vi "Musicplayerversuch_mit_Liste.vi"() -> ()   [LabVIEW 2010]
uses:
  <vilib>/sound2/lvsound2.llb/Sound File Position.ctl
  <vilib>/sound2/lvsound2.llb/Sampling Mode.ctl
  <vilib>/Utility/miscctls.llb/LVRowAndColumnTypeDef.ctl
  <vilib>/Utility/cursorutil.llb/Set Cursor (Icon Pict).vi
  <vilib>/gmath/NI_Gmath.lvlib
  <vilib>/Utility/miscctls.llb/LVKeyTypeDef.ctl
  <vilib>/gmath/statdist.llb/Uniform (Discrete) Random.vi
  <vilib>/Utility/inputDevices.llb/closeKeyboard.vi
  <vilib>/Utility/inputDevices.llb/keyboardAcquire.vi
  <vilib>/sound2/lvsound2.llb/Sound File Read Open.vi
  <vilib>/sound2/lvsound2.llb/Sound File Info (path).vi
  <vilib>/sound2/lvsound2.llb/Sound Output Write (DBL).vi
  <vilib>/sound2/lvsound2.llb/Sound Output Set Volume (Single).vi
  <vilib>/sound2/lvsound2.llb/Sound File Read (DBL).vi
  <vilib>/Utility/file.llb/Write To Spreadsheet File (string).vi
  <vilib>/Utility/file.llb/Read From Spreadsheet File (string).vi
panel:
  in  "plalist umschalten":bool
  in  "Playlist 2":i32(listbox) caption="Playlist"
  in  "nach diesem lied stoppen":bool caption="nach diesem Titel stoppen"
  out "Lieder:":dbl
  in  "shortcut's":bool caption="Kürzel"
  in  "min.Sound":bool caption="min.Lautstärke"
  in  "max.Sound":bool caption="max.Lautsärke"
  in  "counter":bool
  in  "Volume":i64(slide) caption="Lautstärke" min=0 max=100 scale=0.0..100.0
  in  "danach Playlist Start":bool
  in  "Einzeiln":bool
  in  "Hinzufügen":bool
  in  "Musicauswählen":bool
  out "Musicanzeige":string
  in  "Deutsch?":bool
  out "ausgewählt":bool
  out "Zeilezumeinfügen":i32
  in  "Playlist 3":string[][](table)
  in  "veränderung":bool
  out "=":dbl
  in  "Farbfeld":u32(colorbox)
  out "Cluster":T1
  in  "zu spielende Lieder:":dbl
  in  "gespielte Lieder:":dbl
  in  "Gespielte Lieder tabelle":string[][](table)
  in  "icon 2":u16(ring) caption="Symbol"
  in  "icon":u16(ring)=13 caption="Symbol"
  out "Fehler (Ausgang)":errorcluster
  in  "go to line?":bool
  in  "Column":i32
  in  "Row":i32
  in  "Pfad":path
  out "Spalte":dbl
  in  "Seite":dbl
  out "Gelesener Pfad":string
  in  "Language":enum32{"Englisch", "German"}(radio)
  in  "optionen":bool
  in  "Sperren":bool
  out "dup path":path
  in  "anaus":bool
  out "Sicherheitsdati":path
  in  "Start?":bool
  in  "OK Passwort":bool
  out "Text":string="Bitte den Aktivierungscode eingeben."
  out "OK-Schaltfläche":bool
  in  "von, bis":bool
  in  "to":dbl=1.0 caption="bis" min=1.0
  in  "from":dbl=1.0 caption="von" min=1.0
  in  "liste löschen":bool
  in  "gehe zur zeile kn.":bool
  in  "gehe zur zeile":dbl=1.0 min=1.0
  in  "Realtime?":bool
  in  "device ID":u32 caption="Device-ID"
  in  "background":bool
  in  "Info":bool
  in  "Hilfe":bool
  in  "Schließen.":bool
  in  "Pause":bool
  in  "Wiederholen":bool
  in  "Stop":bool
  in  "Play":bool
  out "Verdekung":bool
  in  "Playlist":string[][](table)
  out "Play?":bool
  in  "playlist laden":bool
  in  "playlist speichern":bool
  out "Einzeiln 2":bool
  in  "nächtes lied":bool
  in  "zufall":bool
  out "Lerrerpad?":bool
  out "end of file?":bool caption="Dateiende?"
  in  "zeile entfernen":bool
  out "Stop?":bool
  in  "Wiederholen?":bool
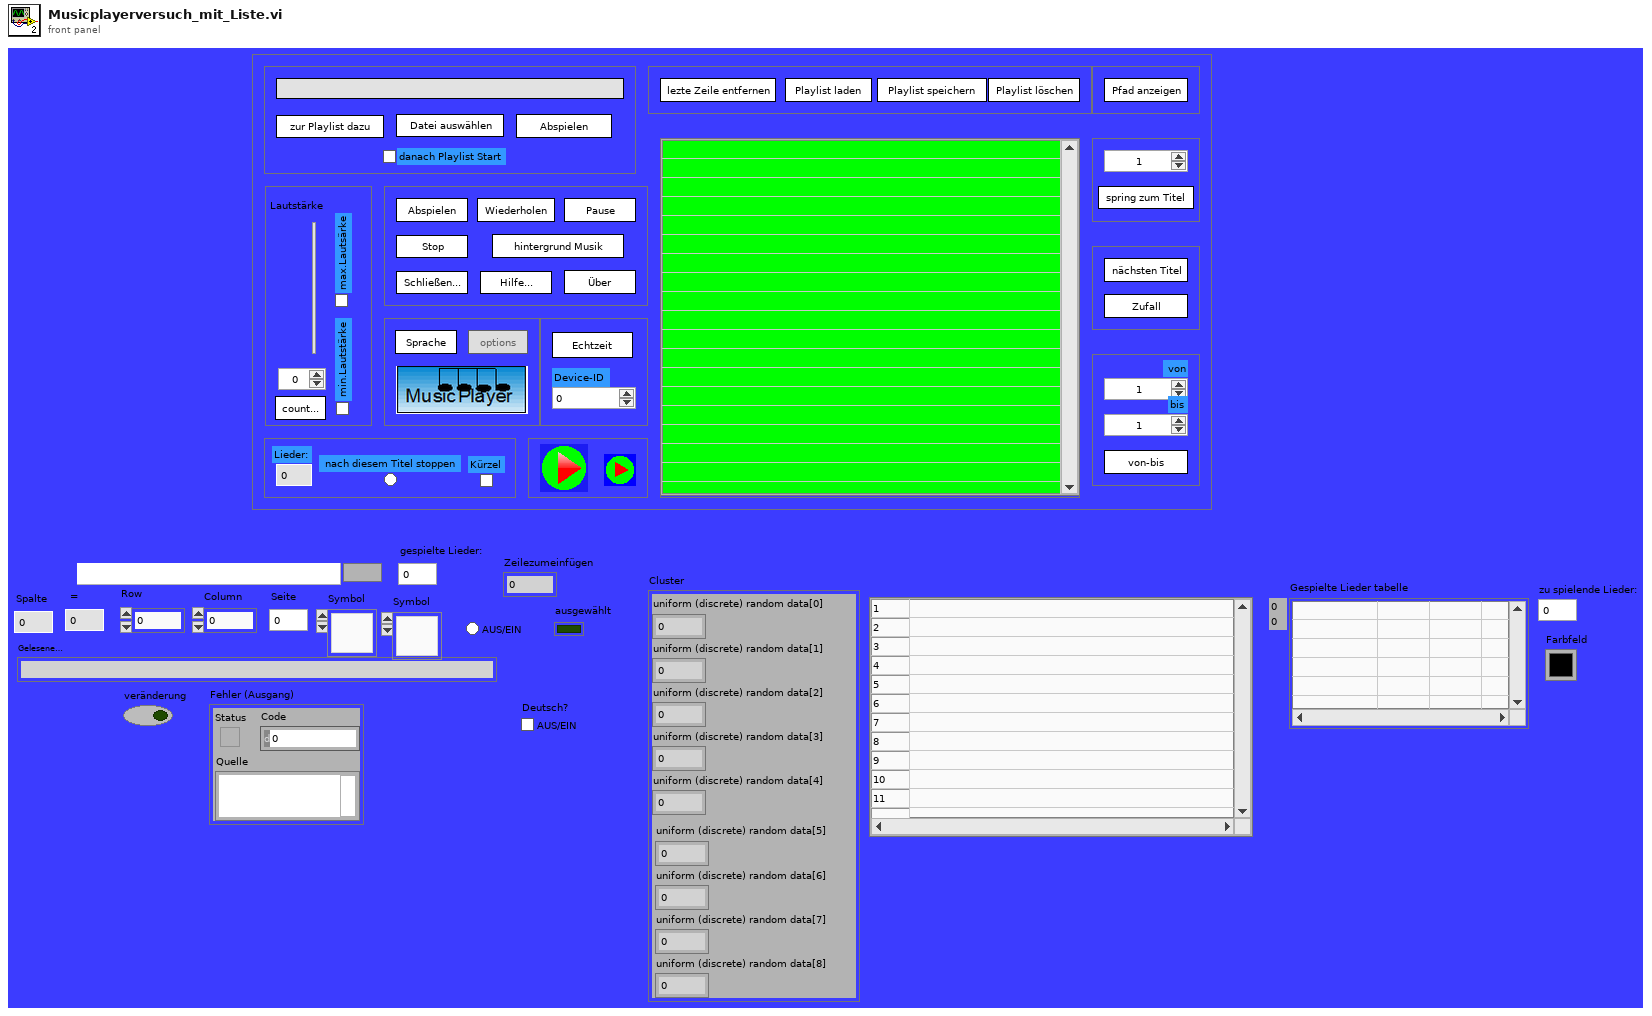
[diagram p1: front panel]
types:
  T1 = cluster{"uniform (discrete) random data[0]":i32, "uniform (discrete) random data[1]":i32, "uniform (discrete) random data[2]":i32, "uniform (discrete) random data[3]":i32, "uniform (discrete) random data[4]":i32, "uniform (discrete) random data[5]":i32, "uniform (discrete) random data[6]":i32, "uniform (discrete) random data[7]":i32, "uniform (discrete) random data[8]":i32}
  T2 = enum16{"open", "replace", "create", "open or create", "replace or create", "replace or create with confirmation"}
  T3 = typedef "LVKeyTypeDef.ctl" = cluster{"Focus":bool, "Control":bool, "Shift":bool, "Key":string}
  T4 = enum16{"0", "1", "2", "3", "4", "5", "6", "7", "8", "9", "A", "B", "C", "D", "E", "F", "G", "H", "I", "J", "K", "L", "M", "N", "O", "P", "Q", "R", "S", "T", "U", "V", "W", "X", "Y", "Z", "F1", "F2", "F3", "F4", "F5", "F6", "F7", "F8", "F9", "F10", "F11", "F12", "F13", "F14", "F15", "ADD", "BACK", "BACKSLASH", "CAPITAL", "COMMA", "DECIMAL", "DELETE", "DIVIDE", "DOWN", "END", "EQUALS", "ESCAPE", "GRAVE (`)", "HOME", "INSERT", "LBRACKET", "LCONTROL", "LEFT", "L ALT", "LSHIFT", "LWIN", "MINUS", "MULTIPLY", "NEXT", "NUMLOCK", "NUMPAD_0", "NUMPAD_1", "NUMPAD_2", "NUMPAD_3", "NUMPAD_4", "NUMPAD_5", "NUMPAD_6", "NUMPAD_7", "NUMPAD_8", "NUMPAD_9", "PAUSE", "PERIOD", "PRIOR (PG UP)", "RBRACKET", "RCONTROL", "RETURN", "RIGHT", "R ALT", "RSHIFT", "RWIN", "SCROLL", "SEMICOLON", "SLASH", "SPACE", "SUBTRACT", "TAB", "UP", "ENTER (num pad)", "' (quote)"}
  T5 = typedef "LVRowAndColumnTypeDef.ctl" = cluster{"Row":i32, "Column":i32}
  T6 = typedef "Sampling Mode.ctl" = i32
  T7 = typedef "Sound Data Format.ctl" = cluster{"sample rate (S/s)":dbl, "number of channels":i32, "bits per sample":i32}
  T8 = typedef "Sound File Refnum.ctl" = refnum<file>
  T9 = typedef "Sound Output Task ID.ctl" = u32
  T10 = typedef "Sound File Position.ctl" = u16
  T11 = enum16{"0", "1", "2", "3", "4", "5", "6", "7", "8", "9", "A", "B", "C", "D", "E", "F", "G", "H", "I", "J", "K", "L", "M", "N", "O", "P", "Q", "R", "S", "T", "U", "V", "W", "X", "Y", "Z", "F1", "F2", "F3", "F4", "F5", "F6", "F7", "F8", "F9", "F10", "F11", "F12", "F13", "F14", "F15", "ADD", "BACK", "BACKSLASH", "CAPITAL", "COMMA", "DECIMAL", "DELETE", "DIVIDE", "DOWN", "END", "EQUALS", "ESCAPE", "GRAVE (`)", "HOME", "INSERT", "LBRACKET", "LCONTROL", "LEFT", "L ALT", "LSHIFT", "LWIN", "MINUS", "MULTIPLY", "NEXT", "NUMLOCK", "NUMPAD_0", "NUMPAD_1", "NUMPAD_2", "NUMPAD_3", "NUMPAD_4", "NUMPAD_5", "NUMPAD_6", "NUMPAD_7", "NUMPAD_8", "NUMPAD_9", "PAUSE", "PERIOD", "PRIOR (PG UP)", "RBRACKET", "RCONTROL", "RETURN", "RIGHT", "R ALT", "RSHIFT", "RWIN", "SCROLL", "SEMICOLON", "SLASH", "SPACE", "SUBTRACT", "TAB", "UP", "ENTER (num pad)", "' (quote)"}[]
  T12 = cluster{"keys pressed[0]":enum16{"0", "1", "2", "3", "4", "5", "6", "7", "8", "9", "A", "B", "C", "D", "E", "F", "G", "H", "I", "J", "K", "L", "M", "N", "O", "P", "Q", "R", "S", "T", "U", "V", "W", "X", "Y", "Z", "F1", "F2", "F3", "F4", "F5", "F6", "F7", "F8", "F9", "F10", "F11", "F12", "F13", "F14", "F15", "ADD", "BACK", "BACKSLASH", "CAPITAL", "COMMA", "DECIMAL", "DELETE", "DIVIDE", "DOWN", "END", "EQUALS", "ESCAPE", "GRAVE (`)", "HOME", "INSERT", "LBRACKET", "LCONTROL", "LEFT", "L ALT", "LSHIFT", "LWIN", "MINUS", "MULTIPLY", "NEXT", "NUMLOCK", "NUMPAD_0", "NUMPAD_1", "NUMPAD_2", "NUMPAD_3", "NUMPAD_4", "NUMPAD_5", "NUMPAD_6", "NUMPAD_7", "NUMPAD_8", "NUMPAD_9", "PAUSE", "PERIOD", "PRIOR (PG UP)", "RBRACKET", "RCONTROL", "RETURN", "RIGHT", "R ALT", "RSHIFT", "RWIN", "SCROLL", "SEMICOLON", "SLASH", "SPACE", "SUBTRACT", "TAB", "UP", "ENTER (num pad)", "' (quote)"}, "keys pressed[1]":enum16{"0", "1", "2", "3", "4", "5", "6", "7", "8", "9", "A", "B", "C", "D", "E", "F", "G", "H", "I", "J", "K", "L", "M", "N", "O", "P", "Q", "R", "S", "T", "U", "V", "W", "X", "Y", "Z", "F1", "F2", "F3", "F4", "F5", "F6", "F7", "F8", "F9", "F10", "F11", "F12", "F13", "F14", "F15", "ADD", "BACK", "BACKSLASH", "CAPITAL", "COMMA", "DECIMAL", "DELETE", "DIVIDE", "DOWN", "END", "EQUALS", "ESCAPE", "GRAVE (`)", "HOME", "INSERT", "LBRACKET", "LCONTROL", "LEFT", "L ALT", "LSHIFT", "LWIN", "MINUS", "MULTIPLY", "NEXT", "NUMLOCK", "NUMPAD_0", "NUMPAD_1", "NUMPAD_2", "NUMPAD_3", "NUMPAD_4", "NUMPAD_5", "NUMPAD_6", "NUMPAD_7", "NUMPAD_8", "NUMPAD_9", "PAUSE", "PERIOD", "PRIOR (PG UP)", "RBRACKET", "RCONTROL", "RETURN", "RIGHT", "R ALT", "RSHIFT", "RWIN", "SCROLL", "SEMICOLON", "SLASH", "SPACE", "SUBTRACT", "TAB", "UP", "ENTER (num pad)", "' (quote)"}, "keys pressed[2]":enum16{"0", "1", "2", "3", "4", "5", "6", "7", "8", "9", "A", "B", "C", "D", "E", "F", "G", "H", "I", "J", "K", "L", "M", "N", "O", "P", "Q", "R", "S", "T", "U", "V", "W", "X", "Y", "Z", "F1", "F2", "F3", "F4", "F5", "F6", "F7", "F8", "F9", "F10", "F11", "F12", "F13", "F14", "F15", "ADD", "BACK", "BACKSLASH", "CAPITAL", "COMMA", "DECIMAL", "DELETE", "DIVIDE", "DOWN", "END", "EQUALS", "ESCAPE", "GRAVE (`)", "HOME", "INSERT", "LBRACKET", "LCONTROL", "LEFT", "L ALT", "LSHIFT", "LWIN", "MINUS", "MULTIPLY", "NEXT", "NUMLOCK", "NUMPAD_0", "NUMPAD_1", "NUMPAD_2", "NUMPAD_3", "NUMPAD_4", "NUMPAD_5", "NUMPAD_6", "NUMPAD_7", "NUMPAD_8", "NUMPAD_9", "PAUSE", "PERIOD", "PRIOR (PG UP)", "RBRACKET", "RCONTROL", "RETURN", "RIGHT", "R ALT", "RSHIFT", "RWIN", "SCROLL", "SEMICOLON", "SLASH", "SPACE", "SUBTRACT", "TAB", "UP", "ENTER (num pad)", "' (quote)"}, "keys pressed[3]":enum16{"0", "1", "2", "3", "4", "5", "6", "7", "8", "9", "A", "B", "C", "D", "E", "F", "G", "H", "I", "J", "K", "L", "M", "N", "O", "P", "Q", "R", "S", "T", "U", "V", "W", "X", "Y", "Z", "F1", "F2", "F3", "F4", "F5", "F6", "F7", "F8", "F9", "F10", "F11", "F12", "F13", "F14", "F15", "ADD", "BACK", "BACKSLASH", "CAPITAL", "COMMA", "DECIMAL", "DELETE", "DIVIDE", "DOWN", "END", "EQUALS", "ESCAPE", "GRAVE (`)", "HOME", "INSERT", "LBRACKET", "LCONTROL", "LEFT", "L ALT", "LSHIFT", "LWIN", "MINUS", "MULTIPLY", "NEXT", "NUMLOCK", "NUMPAD_0", "NUMPAD_1", "NUMPAD_2", "NUMPAD_3", "NUMPAD_4", "NUMPAD_5", "NUMPAD_6", "NUMPAD_7", "NUMPAD_8", "NUMPAD_9", "PAUSE", "PERIOD", "PRIOR (PG UP)", "RBRACKET", "RCONTROL", "RETURN", "RIGHT", "R ALT", "RSHIFT", "RWIN", "SCROLL", "SEMICOLON", "SLASH", "SPACE", "SUBTRACT", "TAB", "UP", "ENTER (num pad)", "' (quote)"}, "keys pressed[4]":enum16{"0", "1", "2", "3", "4", "5", "6", "7", "8", "9", "A", "B", "C", "D", "E", "F", "G", "H", "I", "J", "K", "L", "M", "N", "O", "P", "Q", "R", "S", "T", "U", "V", "W", "X", "Y", "Z", "F1", "F2", "F3", "F4", "F5", "F6", "F7", "F8", "F9", "F10", "F11", "F12", "F13", "F14", "F15", "ADD", "BACK", "BACKSLASH", "CAPITAL", "COMMA", "DECIMAL", "DELETE", "DIVIDE", "DOWN", "END", "EQUALS", "ESCAPE", "GRAVE (`)", "HOME", "INSERT", "LBRACKET", "LCONTROL", "LEFT", "L ALT", "LSHIFT", "LWIN", "MINUS", "MULTIPLY", "NEXT", "NUMLOCK", "NUMPAD_0", "NUMPAD_1", "NUMPAD_2", "NUMPAD_3", "NUMPAD_4", "NUMPAD_5", "NUMPAD_6", "NUMPAD_7", "NUMPAD_8", "NUMPAD_9", "PAUSE", "PERIOD", "PRIOR (PG UP)", "RBRACKET", "RCONTROL", "RETURN", "RIGHT", "R ALT", "RSHIFT", "RWIN", "SCROLL", "SEMICOLON", "SLASH", "SPACE", "SUBTRACT", "TAB", "UP", "ENTER (num pad)", "' (quote)"}, "keys pressed[5]":enum16{"0", "1", "2", "3", "4", "5", "6", "7", "8", "9", "A", "B", "C", "D", "E", "F", "G", "H", "I", "J", "K", "L", "M", "N", "O", "P", "Q", "R", "S", "T", "U", "V", "W", "X", "Y", "Z", "F1", "F2", "F3", "F4", "F5", "F6", "F7", "F8", "F9", "F10", "F11", "F12", "F13", "F14", "F15", "ADD", "BACK", "BACKSLASH", "CAPITAL", "COMMA", "DECIMAL", "DELETE", "DIVIDE", "DOWN", "END", "EQUALS", "ESCAPE", "GRAVE (`)", "HOME", "INSERT", "LBRACKET", "LCONTROL", "LEFT", "L ALT", "LSHIFT", "LWIN", "MINUS", "MULTIPLY", "NEXT", "NUMLOCK", "NUMPAD_0", "NUMPAD_1", "NUMPAD_2", "NUMPAD_3", "NUMPAD_4", "NUMPAD_5", "NUMPAD_6", "NUMPAD_7", "NUMPAD_8", "NUMPAD_9", "PAUSE", "PERIOD", "PRIOR (PG UP)", "RBRACKET", "RCONTROL", "RETURN", "RIGHT", "R ALT", "RSHIFT", "RWIN", "SCROLL", "SEMICOLON", "SLASH", "SPACE", "SUBTRACT", "TAB", "UP", "ENTER (num pad)", "' (quote)"}, "keys pressed[6]":enum16{"0", "1", "2", "3", "4", "5", "6", "7", "8", "9", "A", "B", "C", "D", "E", "F", "G", "H", "I", "J", "K", "L", "M", "N", "O", "P", "Q", "R", "S", "T", "U", "V", "W", "X", "Y", "Z", "F1", "F2", "F3", "F4", "F5", "F6", "F7", "F8", "F9", "F10", "F11", "F12", "F13", "F14", "F15", "ADD", "BACK", "BACKSLASH", "CAPITAL", "COMMA", "DECIMAL", "DELETE", "DIVIDE", "DOWN", "END", "EQUALS", "ESCAPE", "GRAVE (`)", "HOME", "INSERT", "LBRACKET", "LCONTROL", "LEFT", "L ALT", "LSHIFT", "LWIN", "MINUS", "MULTIPLY", "NEXT", "NUMLOCK", "NUMPAD_0", "NUMPAD_1", "NUMPAD_2", "NUMPAD_3", "NUMPAD_4", "NUMPAD_5", "NUMPAD_6", "NUMPAD_7", "NUMPAD_8", "NUMPAD_9", "PAUSE", "PERIOD", "PRIOR (PG UP)", "RBRACKET", "RCONTROL", "RETURN", "RIGHT", "R ALT", "RSHIFT", "RWIN", "SCROLL", "SEMICOLON", "SLASH", "SPACE", "SUBTRACT", "TAB", "UP", "ENTER (num pad)", "' (quote)"}, "keys pressed[7]":enum16{"0", "1", "2", "3", "4", "5", "6", "7", "8", "9", "A", "B", "C", "D", "E", "F", "G", "H", "I", "J", "K", "L", "M", "N", "O", "P", "Q", "R", "S", "T", "U", "V", "W", "X", "Y", "Z", "F1", "F2", "F3", "F4", "F5", "F6", "F7", "F8", "F9", "F10", "F11", "F12", "F13", "F14", "F15", "ADD", "BACK", "BACKSLASH", "CAPITAL", "COMMA", "DECIMAL", "DELETE", "DIVIDE", "DOWN", "END", "EQUALS", "ESCAPE", "GRAVE (`)", "HOME", "INSERT", "LBRACKET", "LCONTROL", "LEFT", "L ALT", "LSHIFT", "LWIN", "MINUS", "MULTIPLY", "NEXT", "NUMLOCK", "NUMPAD_0", "NUMPAD_1", "NUMPAD_2", "NUMPAD_3", "NUMPAD_4", "NUMPAD_5", "NUMPAD_6", "NUMPAD_7", "NUMPAD_8", "NUMPAD_9", "PAUSE", "PERIOD", "PRIOR (PG UP)", "RBRACKET", "RCONTROL", "RETURN", "RIGHT", "R ALT", "RSHIFT", "RWIN", "SCROLL", "SEMICOLON", "SLASH", "SPACE", "SUBTRACT", "TAB", "UP", "ENTER (num pad)", "' (quote)"}, "keys pressed[8]":enum16{"0", "1", "2", "3", "4", "5", "6", "7", "8", "9", "A", "B", "C", "D", "E", "F", "G", "H", "I", "J", "K", "L", "M", "N", "O", "P", "Q", "R", "S", "T", "U", "V", "W", "X", "Y", "Z", "F1", "F2", "F3", "F4", "F5", "F6", "F7", "F8", "F9", "F10", "F11", "F12", "F13", "F14", "F15", "ADD", "BACK", "BACKSLASH", "CAPITAL", "COMMA", "DECIMAL", "DELETE", "DIVIDE", "DOWN", "END", "EQUALS", "ESCAPE", "GRAVE (`)", "HOME", "INSERT", "LBRACKET", "LCONTROL", "LEFT", "L ALT", "LSHIFT", "LWIN", "MINUS", "MULTIPLY", "NEXT", "NUMLOCK", "NUMPAD_0", "NUMPAD_1", "NUMPAD_2", "NUMPAD_3", "NUMPAD_4", "NUMPAD_5", "NUMPAD_6", "NUMPAD_7", "NUMPAD_8", "NUMPAD_9", "PAUSE", "PERIOD", "PRIOR (PG UP)", "RBRACKET", "RCONTROL", "RETURN", "RIGHT", "R ALT", "RSHIFT", "RWIN", "SCROLL", "SEMICOLON", "SLASH", "SPACE", "SUBTRACT", "TAB", "UP", "ENTER (num pad)", "' (quote)"}}
  T13 = enum16{"Left Button", "Center Button", "Right Button", "Window Close"}
  T14 = typedef "eventvkey.ctl" = enum16{"ASCII", "Enter", "Return", "Shift", "Ctrl", "Alt", "Cmd", "Opt", "Caps", "NumLock", "Clear", "Break", "Up", "Down", "Left", "Right", "Insert", "Delete", "Home", "End", "PageUp", "PageDown", "Escape", "Help", "Pause", "ScrollLock", "F1", "F2", "F3", "F4", "F5", "F6", "F7", "F8", "F9", "F10", "F11", "F12", "F13", "F14", "F15", "F16", "F17", "F18", "F19", "F20", "F21", "F22", "F23", "F24", "Play", "VolumeUp", "VolumeDown", "Mute", "Two Byte Char"}
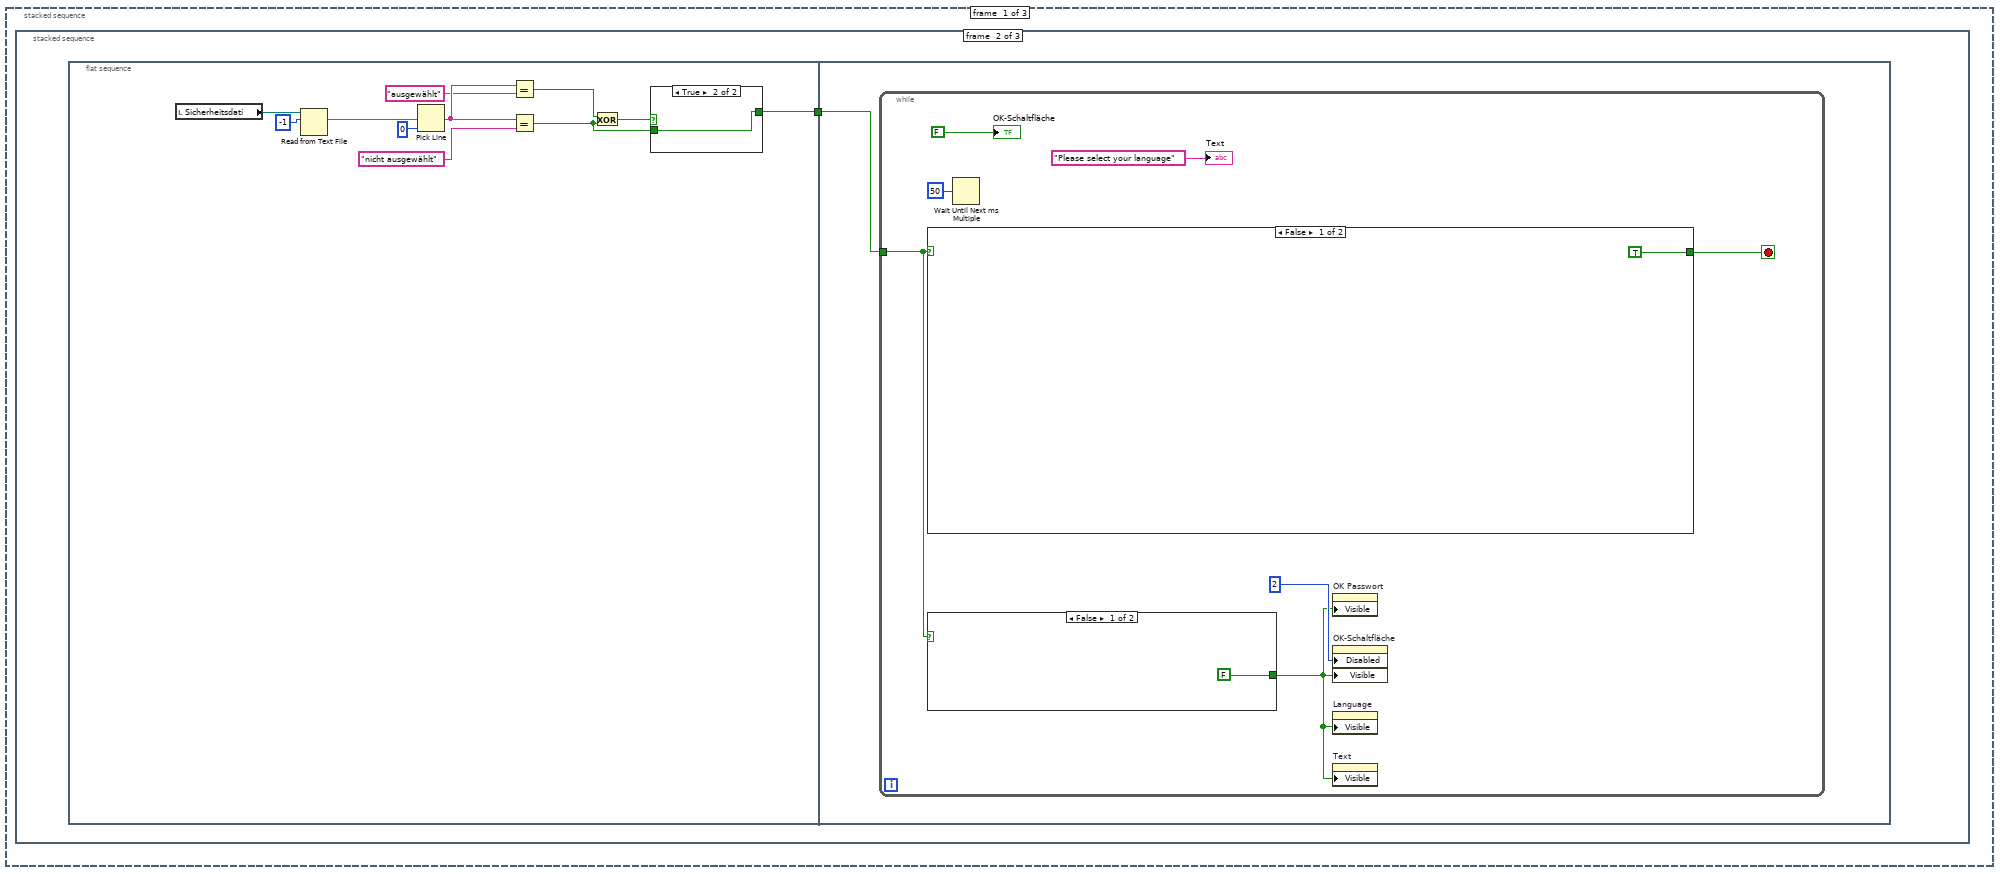
[diagram p2: hidden frame]
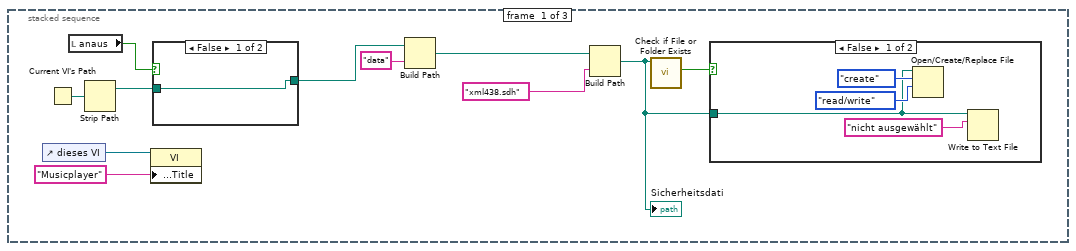
[diagram p3: hidden frame]
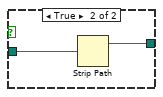
[diagram p4: hidden frame]
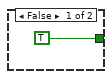
[diagram p6: hidden frame]
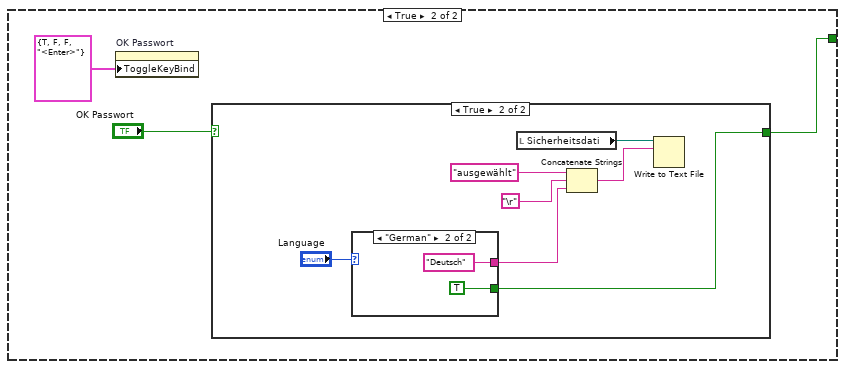
[diagram p7: hidden frame]
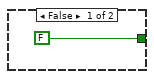
[diagram p8: hidden frame]
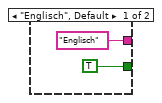
[diagram p9: hidden frame]
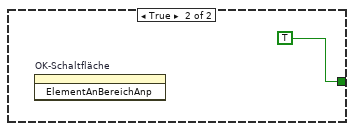
[diagram p10: hidden frame]
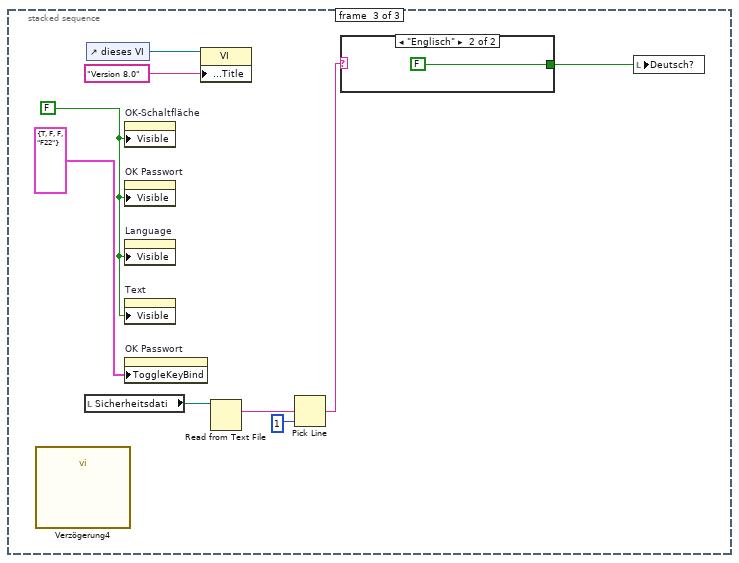
[diagram p11: hidden frame]
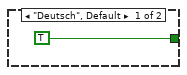
[diagram p12: hidden frame]
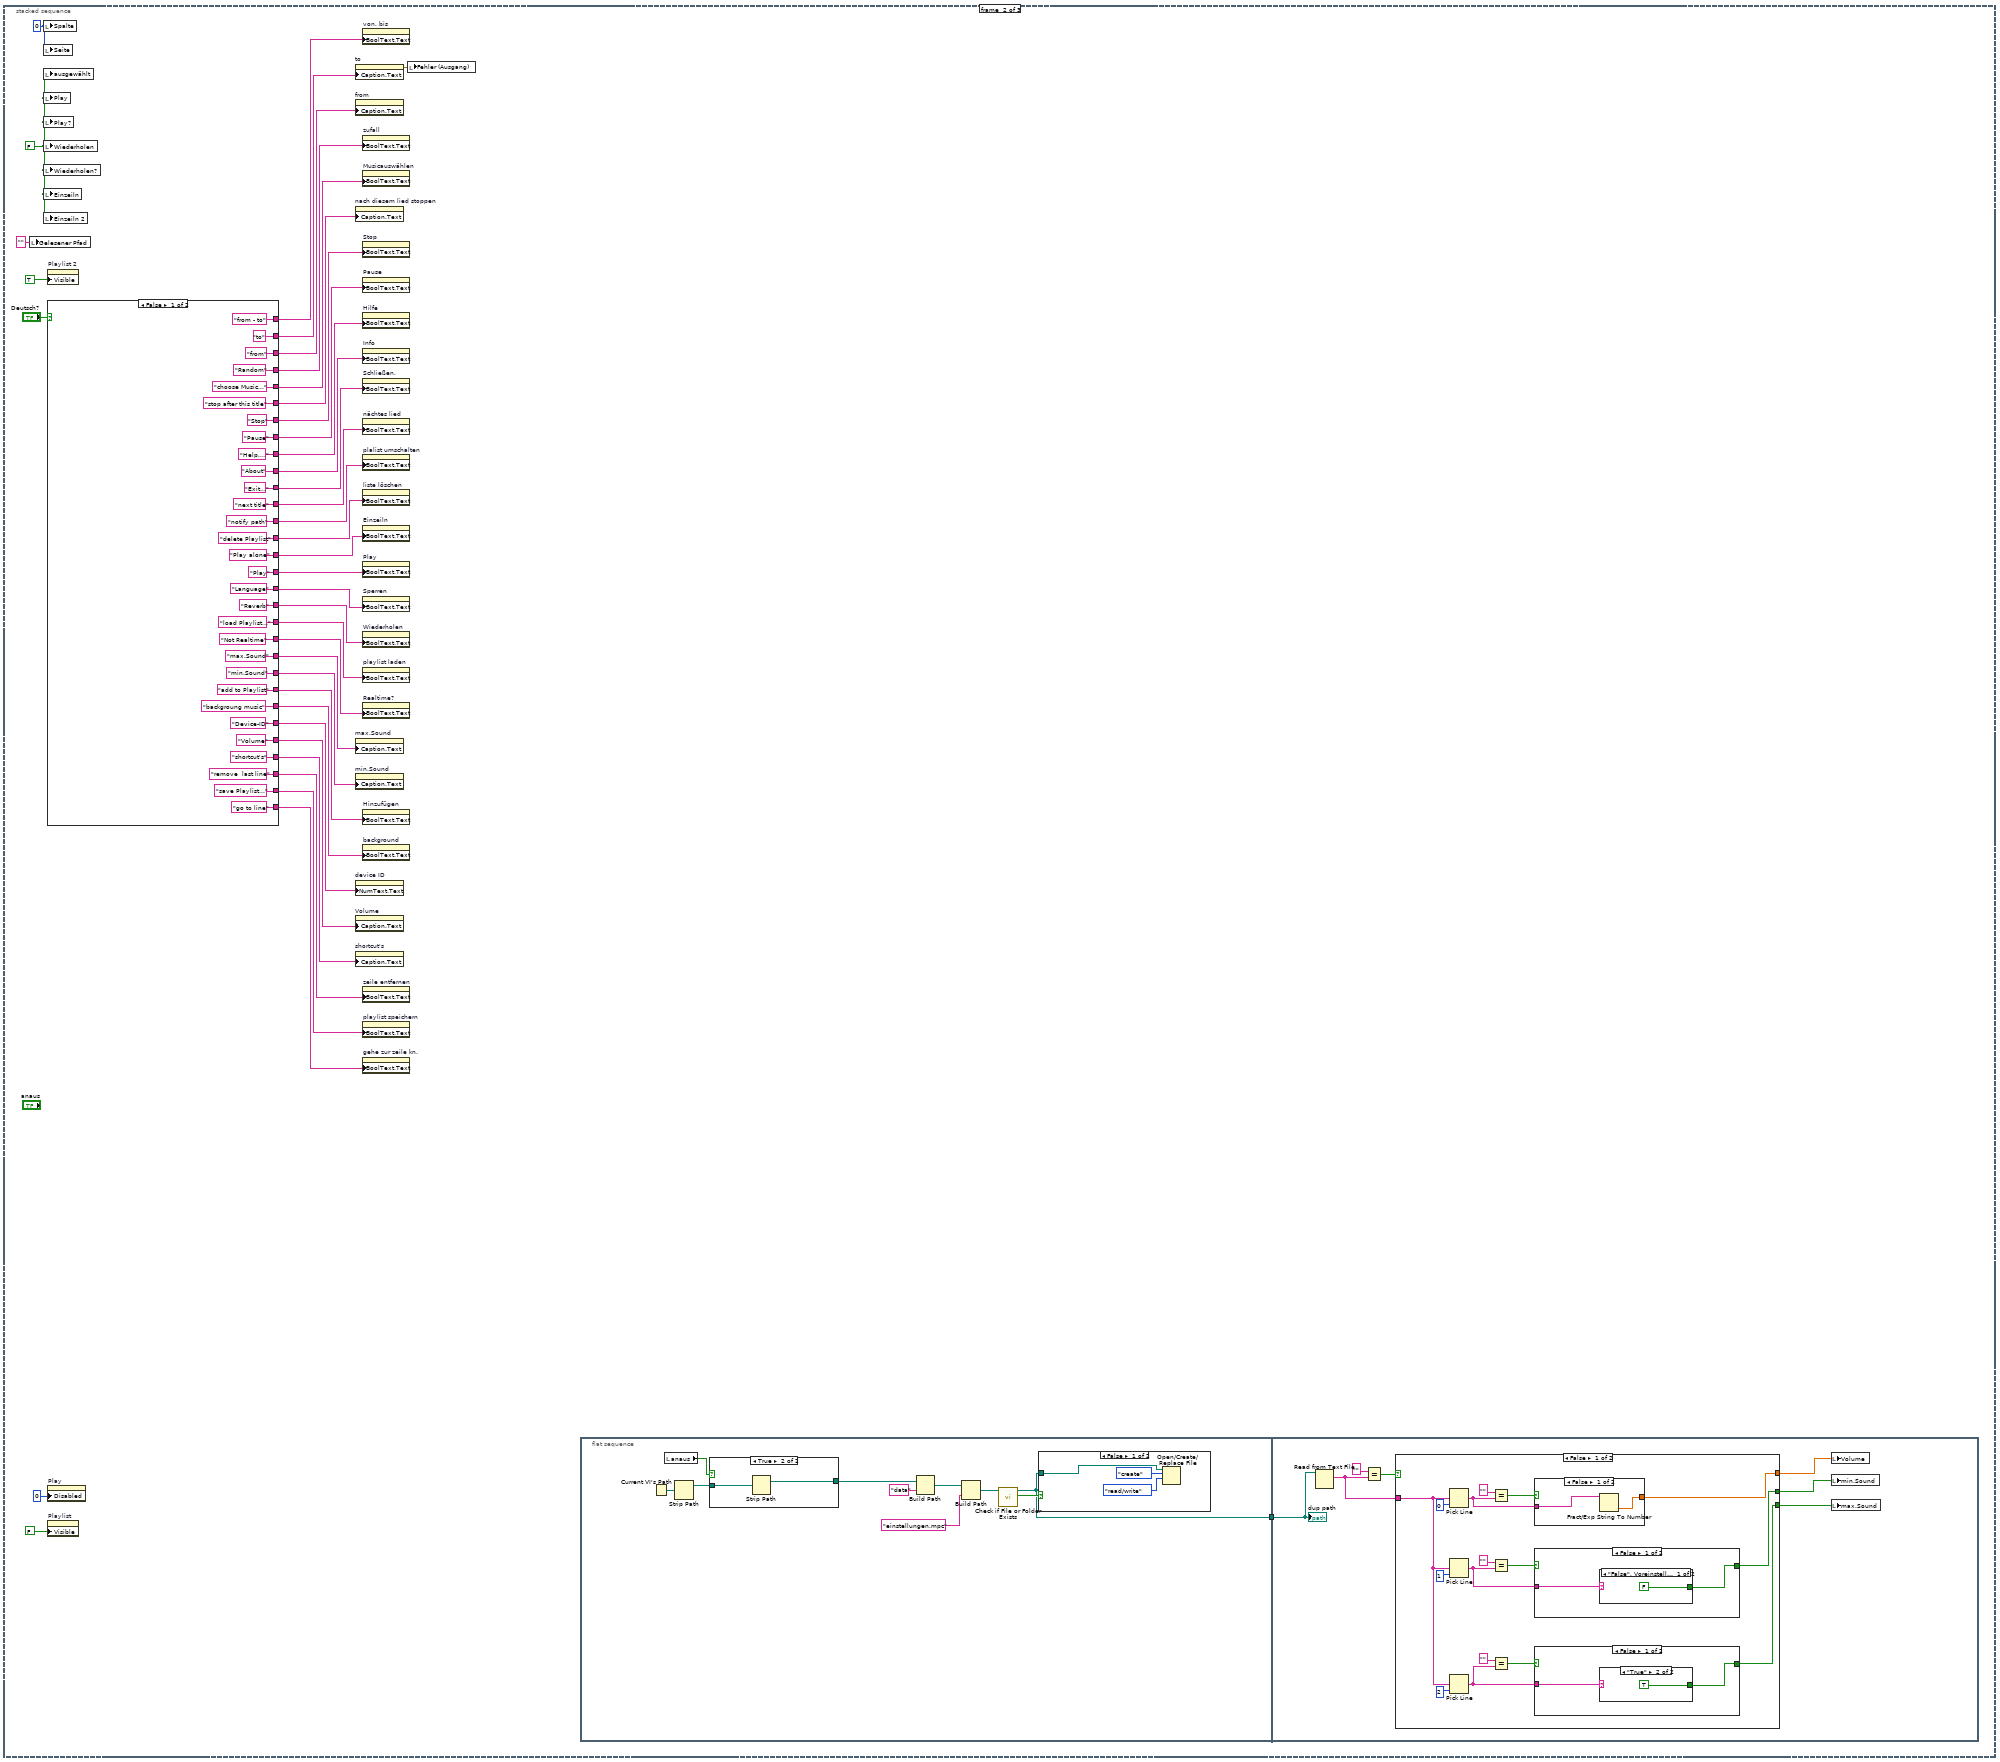
[diagram p13: hidden frame]
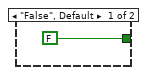
[diagram p16: hidden frame]
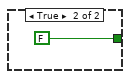
[diagram p17: hidden frame]
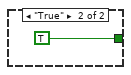
[diagram p18: hidden frame]
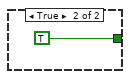
[diagram p19: hidden frame]
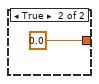
[diagram p20: hidden frame]
diagram:
  # "When you do an Applacion witch this File, than make \"anaus\" true!!!\nElse make \"anaus\" false!!!"
  n1 = stacked-sequence {
    frame #0 {
      n2 = stacked-sequence {
        frame #0 {
          n3 = control-ref of="dieses VI"() -> (w12:refnum<vi>)
          n4 = Current VI's Path() -> (path=w3:path)
          n5 = local read "anaus"() -> (w2:bool)
          n6 = Strip Path(path=w3) -> (stripped path=w8:path)  [unwired: 1 out]
          n7 = property class="VI"(reference=w12, "Front Panel.Title"="Musicplayer") -> ()  [unwired: 1 in, 2 out]
          n8 = case shown="FALSE" w2 {
            tunnel: w8 -> [w13 w15]
            tunnel: [w13 w14] -> w9
            frame False {
            }
            frame True {
              n9 = Strip Path(path=w15) -> (stripped path=w14:path)  [unwired: 1 out]
            }
          }
          n10 = Build Path(base path=w9, name or relative path="data" ("Name oder relativer Pfad")) -> (appended path=w7:path)
          n11 = Build Path(base path=w7, name or relative path="xml438.sdh" ("Name oder relativer Pfad")) -> (appended path=w10:path)
          "Sicherheitsdati" <- w10
          n12 = call <vilib>:"Check if File or Folder Exists.vi"("path"=w10) -> ("file or folder exists?"=w5:bool)  [unwired: 1 in, 9 out]
          n13 = case shown="FALSE" w5 {
            tunnel: w10 -> [w17 _]
            frame False {
              n14 = Open/Create/Replace File(file path (use dialog)=w17, operation (0:open)=T2."create" ("Operation (0:Öffnen)"), access (0:read/write)=enum16{"read/write", "read-only", "write-only"}."read/write" ("Zugriff (0:Lesen/Schreiben)")) -> ()  [unwired: 1 in, 5 out]
              n15 = Write to Text File(file (use dialog)=w17, text="nicht ausgewählt" ("Text")) -> ()  [unwired: 1 in, 4 out]
            }
            frame True {
            }
          }
        }
        frame #1 {
          n16 = flat-sequence {
            tunnel: [w21] -> w20
            tunnel: w20 -> [w34]
            frame #0 {
              n17 = local read "Sicherheitsdati"() -> (w31:path)
              n18 = Read from Text File(file (use dialog)=w31, count=-1 ("Anzahl Bytes (1)")) -> (text=w30:string)  [unwired: 1 in, 4 out]
              n19 = Pick Line(multi-line string=w30, line index=0 ("Zeilenindex")) -> (output string=w29:string)  [unwired: 1 out]
              n20 = Equal?(x=w29, y="ausgewählt") -> (x = y?=w25:bool)
              n21 = Equal?(x=w29, y="nicht ausgewählt") -> (x = y?=w27:bool)
              n22 = Exclusive Or(1:w27, 2:w25) -> (0:w26:bool)
              n23 = case shown="TRUE" w26 {
                tunnel: [TRUE w33] -> w21
                tunnel: w27 -> [_ w33]
                frame False {
                }
                frame True {
                }
              }
            }
            frame #1 {
              n24 = while {
                tunnel: w34 -> [w36]
                stop <- w39 stop-if-true
                n25 = case shown="FALSE" w36 {
                  tunnel: [TRUE w44] -> w39
                  frame False {
                  }
                  frame True {
                    n26 = property on="OK Passwort" class="Bool."("ToggleKeyBind"=T3 {"Focus"=TRUE, "Control"=FALSE, "Shift"=FALSE, "Key"="<Enter>"} ("Umschalttaste")) -> ()  [unwired: 2 in, 2 out]
                    n27 = case shown="TRUE" "OK Passwort" {
                      tunnel: [FALSE w53] -> w44
                      frame False {
                      }
                      frame True {
                        n28 = case shown="\"German\"" "Language" {
                          tunnel: [TRUE TRUE] -> w53
                          tunnel: ["Englisch" "Deutsch"] -> w48
                          frame "Englisch", Default {
                          }
                          frame "German" {
                          }
                        }
                        n29 = local read "Sicherheitsdati"() -> (w47:path)
                        n30 = Concatenate Strings("ausgewählt", "\r", w48) -> (w50:string)
                        n31 = Write to Text File(file (use dialog)=w47, text=w50) -> ()  [unwired: 1 in, 4 out]
                      }
                    }
                  }
                }
                n32 = case shown="FALSE" w36 {
                  tunnel: [FALSE TRUE] -> w35
                  frame False {
                  }
                  frame True {
                    n33 = invoke on="OK-Schaltfläche" class="Boolesch" method="ElementAnBereichAnp"() -> ()  [unwired: 3 in, 3 out]
                  }
                }
                n34 = Wait Until Next ms Multiple(millisecond multiple=50) -> ()  [unwired: 1 out]
                n35 = property on="OK Passwort" class="Bool."("Visible"=w35) -> ()  [unwired: 2 in, 2 out]
                n36 = property on="OK-Schaltfläche" class="Bool."("Disabled"=u8 2 ("Deaktiviert"), "Visible"=w35) -> ()  [unwired: 2 in, 2 out]
                n37 = property on="Language" class="OptionsfelderElem (strikt)"("Visible"=w35) -> ()  [unwired: 2 in, 2 out]
                n38 = property on="Text" class="Str"("Visible"=w35) -> ()  [unwired: 2 in, 2 out]
                "Text" <- "Please select your language"
                "OK-Schaltfläche" <- FALSE
              }
            }
          }
        }
        frame #2 {
          w65 = FALSE
          n39 = call "Verzögerung4"() -> ()  [unwired: 2 in, 10 out]
          n40 = local read "Sicherheitsdati"() -> (w61:path)
          n41 = control-ref of="dieses VI"() -> (w68:refnum<vi>)
          n42 = property on="OK-Schaltfläche" class="Bool."("Visible"=w65) -> ()  [unwired: 2 in, 2 out]
          n43 = property on="OK Passwort" class="Bool."("Visible"=w65) -> ()  [unwired: 2 in, 2 out]
          n44 = property on="Language" class="OptionsfelderElem (strikt)"("Visible"=w65) -> ()  [unwired: 2 in, 2 out]
          n45 = property on="Text" class="Str"("Visible"=w65) -> ()  [unwired: 2 in, 2 out]
          n46 = property on="OK Passwort" class="Bool."("ToggleKeyBind"=T3 {"Focus"=TRUE, "Control"=FALSE, "Shift"=FALSE, "Key"="F22"} ("Umschalttaste")) -> ()  [unwired: 2 in, 2 out]
          n47 = property class="VI"(reference=w68, "Front Panel.Title"="Version 8.0") -> ()  [unwired: 1 in, 2 out]
          n48 = Read from Text File(file (use dialog)=w61) -> (text=w62:string)  [unwired: 1 in, 5 out]
          n49 = Pick Line(multi-line string=w62, line index=1 ("Zeilenindex")) -> (output string=w64:string)  [unwired: 1 out]
          n50 = case shown="\"Englisch\"" w64 {
            tunnel: [TRUE FALSE] -> w60
            frame "Deutsch", Default {
            }
            frame "Englisch" {
            }
          }
          n51 = local write "Deutsch?"(w60) -> ()
        }
      }
    }
    frame #1 {
      w107 = 0
      w72 = FALSE
      n52 = local write "Gelesener Pfad"("") -> ()
      n53 = local write "Spalte"(w107) -> ()
      n54 = local write "Seite"(w107) -> ()
      n55 = local write "ausgewählt"(w72) -> ()
      n56 = local write "Play"(w72) -> ()
      n57 = local write "Play?"(w72) -> ()
      n58 = local write "Wiederholen"(w72) -> ()
      n59 = local write "Wiederholen?"(w72) -> ()
      n60 = local write "Einzeiln"(w72) -> ()
      n61 = local write "Einzeiln 2"(w72) -> ()
      n62 = property on="Playlist 2" class="Listenfeld (strikt)"("Visible"=TRUE) -> ()  [unwired: 2 in, 2 out]
      n63 = case shown="FALSE" "Deutsch?" {
        tunnel: ["next title" ("Boolescher Text.Text") "nächsten Titel" ("Boolescher Text.Text")] -> w104
        tunnel: ["add to Playlist" "zur Playlist dazu"] -> w103
        tunnel: ["choose Music..." ("Boolescher Text.Text") "Datei auswählen" ("Boolescher Text.Text")] -> w102
        tunnel: ["Play alone" "Abspielen"] -> w101
        tunnel: ["Not Realtime" "Echtzeit"] -> w100
        tunnel: ["Language" "Sprache"] -> w99
        tunnel: ["Play" "Abspielen"] -> w98
        tunnel: ["Reverb" "Wiederholen"] -> w97
        tunnel: ["Pause" "Pause"] -> w96
        tunnel: ["Stop" "Stop"] -> w95
        tunnel: ["backgroung music" "hintergrund Musik"] -> w94
        tunnel: ["Exit..." "Schließen..."] -> w93
        tunnel: ["Help...." "Hilfe..."] -> w92
        tunnel: ["About" "Über"] -> w91
        tunnel: ["stop after this title" "nach diesem Titel stoppen"] -> w90
        tunnel: ["Device-ID" "device-nummer"] -> w89
        tunnel: ["max.Sound" "max.Lautsärke"] -> w88
        tunnel: ["min.Sound" "min.Lautstärke"] -> w87
        tunnel: ["shortcut's" "Kürzel"] -> w86
        tunnel: ["from - to" "von-bis"] -> w85
        tunnel: ["to" "bis"] -> w84
        tunnel: ["from" "von"] -> w83
        tunnel: ["Random" "Zufall"] -> w82
        tunnel: ["remove  last line" "lezte Zeile entfernen"] -> w81
        tunnel: ["load Playlist..." "Playlist laden"] -> w80
        tunnel: ["save Playlist..." "Playlist speichern"] -> w79
        tunnel: ["delete Playlist" "Playlist löschen"] -> w78
        tunnel: ["notify path" "Pfad anzeigen"] -> w77
        tunnel: ["go to line" "spring zum Titel"] -> w76
        tunnel: ["Volume" "Lautstärke"] -> w74
        frame False {
        }
        frame True {
        }
      }
      n64 = property on="Play" class="Bool. (strikt)"("Disabled"=0) -> ()  [unwired: 2 in, 2 out]
      n65 = property on="Playlist" class="Tbl (strikt)"("Visible"=FALSE) -> ()  [unwired: 2 in, 2 out]
      n66 = property on="to" class="DigWert (strikt)"("Caption.Text"=w84) -> (error out=w73:errorcluster)  [unwired: 2 in, 1 out]
      n67 = property on="from" class="DigWert (strikt)"("Caption.Text"=w83) -> ()  [unwired: 2 in, 2 out]
      n68 = property on="nach diesem lied stoppen" class="Bool. (strikt)"("Caption.Text"=w90) -> ()  [unwired: 2 in, 2 out]
      n69 = property on="max.Sound" class="Bool. (strikt)"("Caption.Text"=w88) -> ()  [unwired: 2 in, 2 out]
      n70 = property on="min.Sound" class="Bool. (strikt)"("Caption.Text"=w87) -> ()  [unwired: 2 in, 2 out]
      n71 = property on="device ID" class="DigWert (strikt)"("NumText.Text"=w89) -> ()  [unwired: 2 in, 2 out]
      n72 = property on="Volume" class="Schieber (strikt)"("Caption.Text"=w74) -> ()  [unwired: 2 in, 2 out]
      n73 = property on="shortcut's" class="Bool. (strikt)"("Caption.Text"=w86) -> ()  [unwired: 2 in, 2 out]
      n74 = property on="von, bis" class="Bool. (strikt)"("BoolText.Text"=w85) -> ()  [unwired: 2 in, 2 out]
      n75 = property on="zufall" class="Bool. (strikt)"("BoolText.Text"=w82) -> ()  [unwired: 2 in, 2 out]
      n76 = property on="Musicauswählen" class="Bool."("BoolText.Text"=w102) -> ()  [unwired: 2 in, 2 out]
      n77 = property on="Stop" class="Bool. (strikt)"("BoolText.Text"=w95) -> ()  [unwired: 2 in, 2 out]
      n78 = property on="Pause" class="Bool. (strikt)"("BoolText.Text"=w96) -> ()  [unwired: 2 in, 2 out]
      n79 = property on="Hilfe" class="Bool."("BoolText.Text"=w92) -> ()  [unwired: 2 in, 2 out]
      n80 = property on="Info" class="Bool."("BoolText.Text"=w91) -> ()  [unwired: 2 in, 2 out]
      n81 = property on="Schließen." class="Bool."("BoolText.Text"=w93) -> ()  [unwired: 2 in, 2 out]
      n82 = property on="nächtes lied" class="Bool. (strikt)"("BoolText.Text"=w104) -> ()  [unwired: 2 in, 2 out]
      n83 = property on="plalist umschalten" class="Bool. (strikt)"("BoolText.Text"=w77) -> ()  [unwired: 2 in, 2 out]
      n84 = property on="liste löschen" class="Bool."("BoolText.Text"=w78) -> ()  [unwired: 2 in, 2 out]
      n85 = property on="Einzeiln" class="Bool. (strikt)"("BoolText.Text"=w101) -> ()  [unwired: 2 in, 2 out]
      n86 = property on="Play" class="Bool. (strikt)"("BoolText.Text"=w98) -> ()  [unwired: 2 in, 2 out]
      n87 = property on="Sperren" class="Bool."("BoolText.Text"=w99) -> ()  [unwired: 2 in, 2 out]
      n88 = property on="Wiederholen" class="Bool. (strikt)"("BoolText.Text"=w97) -> ()  [unwired: 2 in, 2 out]
      n89 = property on="playlist laden" class="Bool."("BoolText.Text"=w80) -> ()  [unwired: 2 in, 2 out]
      n90 = property on="Realtime?" class="Bool. (strikt)"("BoolText.Text"=w100) -> ()  [unwired: 2 in, 2 out]
      n91 = property on="Hinzufügen" class="Bool."("BoolText.Text"=w103) -> ()  [unwired: 2 in, 2 out]
      n92 = property on="background" class="Bool. (strikt)"("BoolText.Text"=w94) -> ()  [unwired: 2 in, 2 out]
      n93 = property on="zeile entfernen" class="Bool."("BoolText.Text"=w81) -> ()  [unwired: 2 in, 2 out]
      n94 = property on="playlist speichern" class="Bool."("BoolText.Text"=w79) -> ()  [unwired: 2 in, 2 out]
      n95 = property on="gehe zur zeile kn." class="Bool."("BoolText.Text"=w76) -> ()  [unwired: 2 in, 2 out]
      n96 = local write "Fehler (Ausgang)"(w73) -> ()
      n97 = flat-sequence {
        tunnel: [w111] -> w71
        tunnel: w71 -> [w132]
        frame #0 {
          n98 = Current VI's Path() -> (path=w119:path)
          n99 = local read "anaus"() -> (w110:bool)
          n100 = Strip Path(path=w119) -> (stripped path=w118:path)  [unwired: 1 out]
          n101 = case shown="TRUE" w110 {
            tunnel: w118 -> [w120 w122]
            tunnel: [w120 w121] -> w117
            frame False {
            }
            frame True {
              n102 = Strip Path(path=w122) -> (stripped path=w121:path)  [unwired: 1 out]
            }
          }
          n103 = Build Path(base path=w117, name or relative path="data") -> (appended path=w115:path)
          n104 = Build Path(base path=w115, name or relative path="einstellungen.mpc") -> (appended path=w113:path)
          n105 = call <vilib>:"Check if File or Folder Exists.vi"("path"=w113) -> ("file or folder exists?"=w112:bool, "dup path"=w111:path)  [unwired: 1 in, 8 out]
          n106 = case shown="FALSE" w112 {
            tunnel: w111 -> [w125 _]
            frame False {
              n107 = Open/Create/Replace File(file path (use dialog)=w125, operation (0:open)=T2."create" ("Operation (0:Öffnen)"), access (0:read/write)=enum16{"read/write", "read-only", "write-only"}."read/write" ("Zugriff (0:Lesen/Schreiben)")) -> ()  [unwired: 1 in, 5 out]
            }
            frame True {
            }
          }
        }
        frame #1 {
          n108 = Read from Text File(file (use dialog)=w132) -> (text=w127:string)  [unwired: 1 in, 5 out]
          n109 = Equal?(x="", y=w127) -> (x = y?=w128:bool)
          n110 = case shown="FALSE" w128 {
            tunnel: [w147 0.0] -> w131
            tunnel: [w139 TRUE] -> w130
            tunnel: w127 -> [w138 _]
            tunnel: [w135 FALSE] -> w129
            frame False {
              n111 = Pick Line(multi-line string=w138, line index=0 ("Zeilenindex")) -> (output string=w140:string)  [unwired: 1 out]
              n112 = Pick Line(multi-line string=w138, line index=1 ("Zeilenindex")) -> (output string=w141:string)  [unwired: 1 out]
              n113 = Pick Line(multi-line string=w138, line index=2 ("Zeilenindex")) -> (output string=w134:string)  [unwired: 1 out]
              n114 = Equal?(x="", y=w140) -> (x = y?=w148:bool)
              n115 = Equal?(x="", y=w141) -> (x = y?=w142:bool)
              n116 = Equal?(x="", y=w134) -> (x = y?=w136:bool)
              n117 = case shown="FALSE" w148 {
                tunnel: [w160 0.0] -> w147
                tunnel: w140 -> [w159 _]
                frame False {
                  n118 = Fract/Exp String To Number(string=w159) -> (number=w160:dbl)  [unwired: 4 out]
                }
                frame True {
                }
              }
              n119 = case shown="FALSE" w142 {
                tunnel: w141 -> [w155 _]
                tunnel: [w154 TRUE] -> w139
                frame False {
                  n120 = case shown="\"False\", Voreinstellung" w155 {
                    tunnel: [FALSE TRUE] -> w154
                    frame "False", Default {
                    }
                    frame "True" {
                    }
                  }
                }
                frame True {
                }
              }
              n121 = case shown="FALSE" w136 {
                tunnel: w134 -> [w150 _]
                tunnel: [w149 FALSE] -> w135
                frame False {
                  n122 = case shown="\"True\"" w150 {
                    tunnel: [FALSE TRUE] -> w149
                    frame "False", Default {
                    }
                    frame "True" {
                    }
                  }
                }
                frame True {
                }
              }
            }
            frame True {
            }
          }
          n123 = local write "Volume"(w131) -> ()
          n124 = local write "min.Sound"(w130) -> ()
          n125 = local write "max.Sound"(w129) -> ()
          "dup path" <- w132
        }
      }
    }
    frame #2 {
      w225 = "                                                                                ******************************\n                                                                                ****Hilfe zu: Musicplayer****\n                                                                                *****************************\n\nAbspielen aus der Playlist:\n\nWählen Sie eine Datei aus und drücken Sie 1 mal auf \nden \"add to Playlist\" Knopf bis der Dateipfad in der Playlist erscheint.\n\nAbspielen einer Datei unabhängig von der Playlist:\n\nWählen Sie eine Datei aus und drücken Sie auf Play alone, sodass die Datei so abgespielt werden, die Pause, Reverb Tasten können im \"Playlist-\" und im \"Play alone modus\" benutzt werden.\n\n--------------------------------------------------------------------------------------------------------------------\n\n\"next title\" ist zum überspringen einer Datei ín der Playlist gedacht.\n\n\"remove last line\" ist zur entfernung der Letzten Zeile.\n\n\"go to line\" ist bei play in der playlist aktiv, damit kann man zu dem lied springen, wo man hin möchte.\n\n\"Play alone\"ist um die Datei die in der auswahl steht aleine, unabhängig von der Playlist abzuapielen.\n\n\"Reverb\"ist um alle in der Playlist befindlichen Dateien zu iederholen, bei \"Play alone\", wird nur diese eine Datei wiederholt.\n\n\"from - to\" ist um die Lieder von from bis to engegeben sind zuwiederholen\n\n\"count\" ist, um von der jetzigen Lauttärkeposition aus nach oben oder unten zu gehen, also zu faden, dies ist aber nur enmpfehlenswert, wenn de Realtime eingeschaltet ist\n\n\"Random\" spielt die Lieder in zufälligerreienfolege ab, die Funktion ist auch bei \"from - to\" benutzbar, spielt aber nur die Lider \"from\" bis \"to\" ab - zufällig Next Titel ist dann auch noch benutzbar, \"go to line\" auch\n\n\"Kürzel\" schaltet die Abkürtzung ein folgende abkürtzungen gibt es:\n               S: Stop, P: Pause, B: background, W: Reverb, R: Play\n\nEs ist möglich, das nich alles funktioniert.\n\nFÜR JEGLICHE SCHÄDEN, DIE VON DER SOFTWARE AUSGEHEN, WIRD NICHT GEHAFTET. "  # ******************************                                                                                 ****Hilfe zu: Musicplayer****                                                                                 *****************************  Abspielen aus der Playlist:  Wählen Sie eine Datei aus und drücken Sie 1 mal auf  den "add to Playlist" Knopf bis der Dateipfad in der Playlist erscheint.  Abspielen einer Datei unabhängig von der Playlist:  Wählen Sie eine Datei aus und drücken Sie auf Play alone, sodass die Datei so abgespielt werden, die Pause, Reverb Tasten können im "Playlist-" und im "Play alone modus" benutzt werden.  --------------------------------------------------------------------------------------------------------------------  "next title" ist zum überspringen einer Datei ín der Playlist gedacht.  "remove last line" ist zur entfernung der Letzten Zeile.  "go to line" ist bei play in der playlist aktiv, damit kann man zu dem lied springen, wo man hin möchte.  "Play alone"ist um die Datei die in der auswahl steht aleine, unabhängig von der Playlist abzuapielen.  "Reverb"ist um alle in der Playlist befindlichen Dateien zu iederholen, bei "Play alone", wird nur diese eine Datei wiederholt.  "from - to" ist um die Lieder von from bis to engegeben sind zuwiederholen  "count" ist, um von der jetzigen Lauttärkeposition aus nach oben oder unten zu gehen, also zu faden, dies ist aber nur enmpfehlenswert, wenn de Realtime eingeschaltet ist  "Random" spielt die Lieder in zufälligerreienfolege ab, die Funktion ist auch bei "from - to" benutzbar, spielt aber nur die Lider "from" bis "to" ab - zufällig Next Titel ist dann auch noch benutzbar, "go to line" auch  "Kürzel" schaltet die Abkürtzung ein folgende abkürtzungen gibt es:                S: Stop, P: Pause, B: background, W: Reverb, R: Play  Es ist möglich, das nich alles funktioniert.  FÜR JEGLICHE SCHÄDEN, DIE VON DER SOFTWARE AUSGEHEN, WIRD NICHT GEHAFTET.
      n126 = while {
        stop <- FALSE stop-if-true
        n127 = event shown="[2] \"ausgewählt\": Wertänderung" {
          selector: _ -> [_ _ _]
          dyn-events: _ -> [_ _ _]
          timeout: _ -> [_ _ _]
          event "gehe zur zeile": Mouse Enter; "gehe zur zeile": Value Change {
            n128 = event-data() -> ()  [unwired: 4 out]
            n129 = stacked-sequence {
              frame #0 {
                n130 = property on="gehe zur zeile kn." class="Bool."("ToggleKeyBind"=T3 {"Focus"=TRUE, "Control"=FALSE, "Shift"=FALSE, "Key"="<Enter>"} ("Umschalttaste")) -> ()  [unwired: 2 in, 2 out]
              }
              frame #1 {
                n131 = call "Verzögerung10"() -> ()  [unwired: 2 in, 10 out]
              }
              frame #2 {
                n132 = property on="gehe zur zeile kn." class="Bool."("ToggleKeyBind"=T3 {"Focus"=TRUE, "Control"=FALSE, "Shift"=FALSE, "Key"="F24"} ("Umschalttaste")) -> ()  [unwired: 2 in, 2 out]
              }
            }
          }
          event "from", "to": Mouse Enter {
            n133 = event-data() -> ()  [unwired: 5 out]
            n134 = stacked-sequence {
              frame #0 {
                n135 = property on="von, bis" class="Bool. (strikt)"("ToggleKeyBind"=T3 {"Focus"=TRUE, "Control"=FALSE, "Shift"=FALSE, "Key"="<Enter>"} ("Umschalttaste")) -> ()  [unwired: 2 in, 2 out]
              }
              frame #1 {
                n136 = call "Verzögerung11"() -> ()  [unwired: 2 in, 10 out]
              }
              frame #2 {
                n137 = property on="von, bis" class="Bool. (strikt)"("ToggleKeyBind"=T3 {"Focus"=TRUE, "Control"=FALSE, "Shift"=FALSE, "Key"="F23"} ("Umschalttaste")) -> ()  [unwired: 2 in, 2 out]
              }
            }
          }
          event "ausgewählt": Value Change {
            n138 = event-data() -> ("NewVal"=w233:bool)  [unwired: 4 out]
            n139 = case shown="TRUE" w233 {
              frame False {
              }
              frame True {
                n140 = stacked-sequence {
                  frame #0 {
                    n141 = local write "ausgewählt"(FALSE) -> ()
                    n142 = property on="Hinzufügen" class="Bool."("ToggleKeyBind"=T3 {"Focus"=TRUE, "Control"=FALSE, "Shift"=FALSE, "Key"="<Enter>"} ("Umschalttaste")) -> ()  [unwired: 2 in, 2 out]
                  }
                  frame #1 {
                    n143 = call "Verzögerung12"() -> ()  [unwired: 2 in, 10 out]
                  }
                  frame #2 {
                    n144 = property on="Hinzufügen" class="Bool."("ToggleKeyBind"=T3 {"Focus"=TRUE, "Control"=FALSE, "Shift"=FALSE, "Key"="F21"} ("Umschalttaste")) -> ()  [unwired: 2 in, 2 out]
                  }
                }
              }
            }
          }
        }
        n145 = Wait Until Next ms Multiple(millisecond multiple=50) -> ()  [unwired: 1 out]
      }
      n146 = while {
        stop <- FALSE stop-if-true
        # "Lieder=10 - from= 5 Y= 5,  to= 7 - Y=5 = 3, X= 3"
        # "Bsp: Lieder= 10, from= 5, to= 7\nLiederzuspielen?= X, X= 3: 5 6 7\n                                               1 2 3"
        # "Lieder - from = X,"
        n147 = local read "Pause"() -> (w688:bool)
        n148 = local read "Play?"() -> (w683:bool)
        n149 = local read "Play?"() -> (w685:bool)
        n150 = local read "Play?"() -> (w691:bool)
        n151 = Wait Until Next ms Multiple(millisecond multiple=50) -> ()  [unwired: 1 out]
        n152 = local read "Einzeiln 2"() -> (w693:bool)
        n153 = local read "Play?"() -> (w689:bool)
        n154 = local read "Stop?"() -> (w698:bool)
        n155 = case shown="TRUE" w683 {
          frame False {
          }
          frame True {
            n156 = local read "von, bis"() -> (w705:bool)
            n157 = case shown="FALSE" w705 {
              tunnel: [w709 w711] -> w703
              frame False {
                n158 = local write "veränderung"(FALSE) -> ()
                n159 = local read "Lieder:"() -> (w709:dbl)
              }
              frame True {
                n160 = case shown="TRUE" "veränderung" {
                  tunnel: [w713 w716] -> w711
                  frame False {
                    n161 = local read "from"() -> (w714:dbl)
                    n162 = local read "to"() -> (w715:dbl)
                    n163 = call "Liederberechnung.vi"("to:"=w715, "from:"=w714) -> ("ende?"=w712:bool, "X:"=w713:dbl)  [unwired: 8 out]
                    "=" <- w713
                    n164 = local write "veränderung"(w712) -> ()
                  }
                  frame True {
                    n165 = local read "="() -> (w716:dbl)
                  }
                }
              }
            }
            n166 = local read "Wiederholen?"() -> (w704:bool)
            n167 = case shown="FALSE" w704 {
              tunnel: w703 -> [w706 _]
              tunnel: [w706 inf] -> w702
              frame False {
              }
              frame True {
              }
            }
            n168 = local write "zu spielende Lieder:"(w702) -> ()
          }
        }
        n169 = case shown="TRUE" w685 {
          tunnel: ["Musicplayer" w722] -> w684
          frame False {
          }
          frame True {
            n170 = local read "Pause"() -> (w723:bool)
            n171 = local read "Gelesener Pfad"() -> (w719:string)
            n172 = case shown="TRUE" w723 {
              tunnel: ["" "-pause-"] -> w721
              frame False {
              }
              frame True {
              }
            }
            n173 = String To Path(string=w719) -> (path=w720:path)
            n174 = call <vilib>:"Get File Extension.vi"("file"=w720) -> ("filename without extension"=w718:string)  [unwired: 1 in, 9 out]
            n175 = Concatenate Strings(w721, w718) -> (w722:string)
          }
        }
        n176 = case shown="TRUE" w691 {
          tunnel: [w729 w733] -> w677
          tunnel: [w729 w734] -> w678
          tunnel: [w729 2] -> w682
          tunnel: [w729 w731] -> w681
          tunnel: [w729 w730] -> w676
          frame False {
            w729 = 0
          }
          frame True {
            n177 = local read "Einzeiln 2"() -> (w735:bool)
            n178 = case shown="FALSE" w735 {
              tunnel: [2 0] -> w734
              tunnel: [w739 2] -> w733
              tunnel: [u32 16711680 ("Farbfeld") u32 16777228 ("Farbfeld")] -> w731
              tunnel: [0 2] -> w730
              frame False {
                n179 = local read "nach diesem lied stoppen"() -> (w737:bool)
                n180 = case shown="TRUE" w737 {
                  frame False {
                  }
                  frame True {
                    w741 = FALSE
                    n181 = local write "nächtes lied"(w741) -> ()
                    n182 = local write "Wiederholen"(w741) -> ()
                    n183 = local write "von, bis"(w741) -> ()
                    n184 = local write "Wiederholen?"(w741) -> ()
                  }
                }
                n185 = case shown="TRUE" w737 {
                  tunnel: [0 2] -> w739
                  frame False {
                  }
                  frame True {
                  }
                }
              }
              frame True {
              }
            }
          }
        }
        n186 = Bundle("Row"="Row", "Column"="Column") -> (w673:cluster{"Row":i32, "Column":i32})  [unwired: 1 out]
        n187 = And(x=w688, y=w689) -> (x .and. y?=w690:bool)
        n188 = Not(x=w698) -> (.not. x?=w694:bool)
        n189 = Not(x=w693) -> (.not. x?=w692:bool)
        n190 = property on="Playlist 2" class="Listenfeld (strikt)"("SelColor"="Farbfeld") -> ()  [unwired: 2 in, 2 out]
        n191 = property on="Playlist" class="Tbl (strikt)"("Selection Color"="Farbfeld", "Selection Size"=T5 {"Row"=1, "Column"=1} ("Größe des markierten Bereichs"), "Selection Start"=w673) -> ()  [unwired: 2 in, 2 out]
        n192 = case shown="FALSE" w690 {
          frame False {
            n193 = call-poly <vilib>:"Set Cursor.vi"("icon"="icon 2") -> ()  [unwired: 2 in, 9 out]
          }
          frame True {
            n194 = call-poly <vilib>:"Set Cursor.vi"("icon"="icon") -> ()  [unwired: 2 in, 9 out]
          }
        }
        n195 = Or(x=w694, y=w692) -> (x .or. y?=w695:bool)
        n196 = local read "Play?"() -> (w699:bool)
        n197 = And(x=w699, y=w695) -> (x .and. y?=w675:bool)
        n198 = case shown="FALSE" w675 {
          tunnel: [w754 TRUE ("Aktive Zelle:Schriftart der Zelle:Fett")] -> w697
          frame False {
            n199 = while {
              tunnel: [FALSE] -> w754
              shift-right: [w757] -> _
              shift-left: 0 -> [w758]
              stop <- w760 stop-if-true
              w755 = FALSE
              n200 = local read "Playlist"() -> (w765:string[][])
              n201 = Wait Until Next ms Multiple(millisecond multiple=50) -> ()  [unwired: 1 out]
              n202 = Index Array(array=w765, index (row)=w758, index (col)=0 ("Deaktivierter Index (Spalte)")) -> (element=w763:string)
              n203 = Equal?(x=w763, y="") -> (x = y?=w762:bool)
              n204 = case shown="FALSE" w762 {
                tunnel: [w769 w772] -> w757
                tunnel: w758 -> [w768 w772]
                tunnel: [FALSE TRUE] -> w760
                frame False {
                  n205 = Increment(x=w768) -> (x+1=w769:i32)
                }
                frame True {
                }
              }
              n206 = Bundle(w757, 0) -> (w756:cluster{i32, i32})  [unwired: 1 out]
              n207 = property on="Playlist 2" class="Listenfeld (strikt)"("Active Row"=w757, "CellFontBold"=w755) -> ()  [unwired: 2 in, 2 out]
              n208 = property on="Playlist" class="Tbl (strikt)"("Active Cell"=w756, "CellFontBold"=w755) -> ()  [unwired: 2 in, 2 out]
            }
          }
          frame True {
          }
        }
        n209 = control-ref of="dieses VI"() -> (w686:refnum<vi>)
        n210 = property class="VI"(reference=w686, "Front Panel.Title"=w684) -> ()  [unwired: 1 in, 2 out]
        n211 = local read "nächtes lied"() -> (w687:bool)
        n212 = local write "Farbfeld"(w681) -> ()
        n213 = property on="device ID" class="DigWert (strikt)"("Disabled"=w682) -> ()  [unwired: 2 in, 2 out]
        n214 = property on="nach diesem lied stoppen" class="Bool. (strikt)"("Disabled"=w676) -> ()  [unwired: 2 in, 2 out]
        n215 = property on="playlist laden" class="Bool."("Disabled"=w678) -> ()  [unwired: 2 in, 2 out]
        n216 = property on="Hinzufügen" class="Bool."("Disabled"=w678) -> ()  [unwired: 2 in, 2 out]
        n217 = case shown="FALSE" w687 {
          tunnel: w677 -> [_ w726]
          frame False {
          }
          frame True {
            n218 = property on="nächtes lied" class="Bool. (strikt)"("Disabled"=w726) -> ()  [unwired: 2 in, 2 out]
          }
        }
        n219 = property on="gehe zur zeile kn." class="Bool."("Disabled"=w677) -> ()  [unwired: 2 in, 2 out]
        n220 = property on="gehe zur zeile" class="DigWert (strikt)"("Disabled"=w677) -> ()  [unwired: 2 in, 2 out]
        n221 = property on="liste löschen" class="Bool."("Disabled"=w678) -> ()  [unwired: 2 in, 2 out]
        n222 = property on="zeile entfernen" class="Bool."("Disabled"=w678) -> ()  [unwired: 2 in, 2 out]
        n223 = property on="von, bis" class="Bool. (strikt)"("Disabled"=w677) -> ()  [unwired: 2 in, 2 out]
        n224 = local read "Spalte"() -> (w696:dbl)
        n225 = local write "Row"(w696) -> ()
        n226 = case shown="TRUE" w675 {
          tunnel: w697 -> [_ _]
          tunnel: w696 -> [_ w748]
          frame False {
          }
          frame True {
            n227 = Bundle("Spalte"=w748, 0) -> (w751:cluster{"Spalte":dbl, i32})  [unwired: 1 out]
            n228 = property on="Playlist 2" class="Listenfeld (strikt)"("Active Row"=w748, "CellFontBold"=TRUE ("Aktive Zeile:Schriftart der Zelle:Fett")) -> ()  [unwired: 2 in, 2 out]
            n229 = property on="Playlist" class="Tbl (strikt)"("CellFontBold"=TRUE ("Aktive Zelle:Schriftart der Zelle:Fett"), "Active Cell"=w751) -> ()  [unwired: 2 in, 2 out]
          }
        }
      }
      n230 = while {
        shift-right: [w1039] -> _
        shift-left: 0 -> [w1038]
        stop <- FALSE stop-if-true
        n231 = Wait Until Next ms Multiple(millisecond multiple=50) -> ()  [unwired: 1 out]
        n232 = Wait Until Next ms Multiple(millisecond multiple=50) -> ()  [unwired: 1 out]
        n233 = local read "Einzeiln 2"() -> (w1037:bool)
        n234 = local write "Wiederholen?"("Wiederholen") -> ()
        n235 = Not(x=w1037) -> (.not. x?=w1033:bool)
        n236 = case shown="TRUE" "playlist laden" {
          frame False {
          }
          frame True {
            n237 = Open/Create/Replace File(prompt="load Playlist" ("Eingabeaufforderung"), operation (0:open)=T2."open" ("Operation (0:Öffnen)"), access (0:read/write)=enum16{"read/write", "read-only", "write-only"}."read/write" ("Zugriff (0:Lesen/Schreiben)")) -> (refnum out=w1047:refnum<file>, cancelled=w1045:bool, error out=→"Fehler (Ausgang)":errorcluster)  [unwired: 1 in, 2 out]
            n238 = case shown="FALSE" w1045 {
              tunnel: w1047 -> [w1051 _]
              frame False {
                n239 = flat-sequence {
                  tunnel: w1051 -> [w1052]
                  tunnel: [w1052] -> w1050
                  tunnel: w1050 -> [w1055]
                  frame #0 {
                    n240 = Refnum to Path(1:w1052) -> (0:w1053:path)
                    n241 = call-poly <vilib>:"Read From Spreadsheet File.vi"("file path (dialog if empty)"=w1053) -> ("all rows"=w1054:string[][])  [unwired: 3 in, 7 out]
                    n242 = local write "Playlist 3"(w1054) -> ()
                  }
                  frame #1 {
                    n243 = Close File(refnum=w1055) -> ()  [unwired: 1 in, 2 out]
                  }
                  frame #2 {
                    n244 = while {
                      shift-right: [w1061] -> _
                      shift-left: 0 -> [w1062]
                      stop <- w1058 stop-if-true
                      n245 = Wait Until Next ms Multiple(millisecond multiple=50) -> ()  [unwired: 1 out]
                      n246 = Index Array(array="Playlist 3", index (row)=w1062, index (col)=0) -> (element=w1059:string)
                      n247 = Equal?(x=w1059, y="") -> (x = y?=w1058:bool)
                      n248 = case shown="FALSE" w1058 {
                        tunnel: w1062 -> [w1074 w1118]
                        tunnel: [w1073 w1118] -> w1061
                        tunnel: w1059 -> [w1068 _]
                        frame False {
                          n249 = String To Path(string=w1068) -> (path=w1072:path)
                          n250 = call <vilib>:"Get File Extension.vi"("file"=w1072) -> ("filename without extension"=w1069:string, "lowercase file extension"=w1067:string)  [unwired: 1 in, 8 out]
                          n251 = Equal?(x=w1067, y="wav") -> (x = y?=w1065:bool)
                          n252 = call <vilib>:"Check if File or Folder Exists.vi"("path"=w1072) -> ("file or folder exists?"=w1066:bool)  [unwired: 1 in, 9 out]
                          n253 = And(x=w1066, y=w1065) -> (x .and. y?=w1070:bool)
                          n254 = case shown="TRUE" w1070 {
                            tunnel: w1074 -> [w1076 w1087]
                            tunnel: [w1079 w1090] -> w1073
                            tunnel: w1069 -> [_ w1088]
                            tunnel: w1068 -> [_ w1086]
                            frame False {
                              n255 = Bundle(w1076, 0) -> (w1081:cluster{i32, i32})  [unwired: 1 out]
                              n256 = property on="Playlist" class="Tbl (strikt)"("Selection Size"=T5 {"Row"=1, "Column"=1} ("Größe des markierten Bereichs"), "Selection Start"=w1081, "Selection Color"=u32 5 ("Markierfarbe")) -> ()  [unwired: 2 in, 2 out]
                              n257 = call "Fehler"() -> ("OK"=w1075:bool)  [unwired: 3 in, 8 out]
                              n258 = case shown="FALSE" w1075 {
                                tunnel: [w1083 w1085] -> w1077
                                tunnel: w1076 -> [w1083 w1084]
                                frame False {
                                }
                                frame True {
                                n259 = Increment(x=w1084) -> (x+1=w1085:i32)
                                }
                              }
                              n260 = Increment(x=w1077) -> (x+1=w1079:i32)
                            }
                            frame True {
                              n261 = stacked-sequence {
                                tunnel: [_ _ _ TRUE] -> w1089
                                tunnel: w1088 -> [_ w1105 _ _]
                                tunnel: w1086 -> [_ _ w1109 _]
                                frame #0 {
                                n262 = while {
                                shift-right: [w1092] -> _
                                shift-left: 0 -> [w1093]
                                stop <- w1094 stop-if-true
                                n263 = local read "Playlist"() -> (w1098:string[][])
                                n264 = Index Array(array=w1098, index (row)=w1093, index (col)=0 ("Deaktivierter Index (Spalte)")) -> (element=w1096:string)
                                n265 = Equal?(x=w1096, y="") -> (x = y?=w1094:bool)
                                n266 = case shown="TRUE" w1094 {
                                tunnel: w1093 -> [w1099 w1101]
                                tunnel: [w1100 w1101] -> w1092
                                frame False {
                                n267 = Increment(x=w1099) -> (x+1=w1100:i32)
                                }
                                frame True {
                                "Zeilezumeinfügen" <- w1101
                                }
                                }
                                }
                                }
                                frame #1 {
                                n268 = property on="Playlist 2" class="Listenfeld (strikt)"() -> ("Item Names"=w1103:string[])  [unwired: 2 in, 2 out]
                                n269 = local read "Zeilezumeinfügen"() -> (w1104:i32)
                                n270 = Initialize Array(w1105, 1 ("Dimension")) -> (w1106:string[])
                                n271 = Insert Into Array(array=w1103, index=w1104, new element=w1106) -> (w1102:string[])
                                n272 = property on="Playlist 2" class="Listenfeld (strikt)"("Item Names"=w1102) -> ()  [unwired: 2 in, 2 out]
                                }
                                frame #2 {
                                n273 = local read "Zeilezumeinfügen"() -> (w1112:i32)
                                n274 = local read "Playlist"() -> (w1113:string[][])
                                n275 = Initialize Array(w1109, 1) -> (w1110:string[])
                                n276 = Insert Into Array(array=w1113, index (row)=w1112, new element=w1110) -> (w1108:string[][])  [unwired: 1 in]
                                n277 = local write "Playlist"(w1108) -> ()
                                }
                                frame #3 {
                                }
                              }
                              n278 = case shown="TRUE" w1089 {
                                tunnel: w1087 -> [w1115 w1117]
                                tunnel: [w1115 w1116] -> w1090
                                frame False {
                                }
                                frame True {
                                n279 = Increment(x=w1117) -> (x+1=w1116:i32)
                                }
                              }
                            }
                          }
                        }
                        frame True {
                        }
                      }
                    }
                  }
                  frame #3 {
                  }
                }
              }
              frame True {
              }
            }
          }
        }
        n280 = local read "Play?"() -> (w1032:bool)
        n281 = And(x=w1033, y=w1032) -> (x .and. y?=w1034:bool)
        n282 = case shown="TRUE" w1034 {
          tunnel: w1038 -> [_ w1124]
          tunnel: [0 w1123] -> w1039
          tunnel: [FALSE TRUE] -> w1040
          frame False {
          }
          frame True {
            n283 = case shown="1" w1124 {
              selector: w1124 -> [w1127 _]
              tunnel: [w1126 0] -> w1123
              tunnel: [TRUE FALSE] -> w1121
              frame 0, Default {
                n284 = call "Verzögerung5"() -> ()  [unwired: 2 in, 10 out]
                n285 = Increment(x=w1127) -> (x+1=w1126:i32)
              }
              frame 1 {
                n286 = call "Verzögerung6"() -> ()  [unwired: 2 in, 10 out]
              }
            }
            "Verdekung" <- w1121
          }
        }
        n287 = property on="Verdekung" class="Bool. (strikt)"("Visible"=w1040) -> ()  [unwired: 2 in, 2 out]
      }
      n288 = while {
        stop <- FALSE stop-if-true
        n289 = Wait Until Next ms Multiple(millisecond multiple=50) -> ()  [unwired: 1 out]
        n290 = property on="gehe zur zeile kn." class="Bool."("Disabled"=0) -> ()  [unwired: 2 in, 2 out]
        n291 = case shown="FALSE" "Einzeiln" {
          frame False {
          }
          frame True {
            "Einzeiln 2" <- TRUE
          }
        }
        n292 = Compound Arithmetic op=OR("Play", "Einzeiln") -> (w239:bool)
        "Play?" <- w239
        n293 = case shown="TRUE" w239 {
          frame False {
            w245 = 0
            w247 = inf
            w244 = FALSE
            w246 = 0
            (unwired) path ""
            n294 = local write "Gelesener Pfad"("") -> ()
            n295 = local write "Einzeiln 2"(w244) -> ()
            n296 = local write "nach diesem lied stoppen"(w244) -> ()
            n297 = local write "end of file?"(w244) -> ()
            n298 = local write "Play?"(w244) -> ()
            n299 = local write "Stop?"(w244) -> ()
            n300 = local write "Stop"(w244) -> ()
            n301 = local write "Lerrerpad?"(w244) -> ()
            n302 = local write "Spalte"(w246) -> ()
            n303 = local write "Seite"(w246) -> ()
            n304 = local write "gespielte Lieder:"(w246) -> ()
            n305 = property on="to" class="DigWert (strikt)"("Maximum"=w247) -> ()  [unwired: 2 in, 2 out]
            n306 = property on="from" class="DigWert (strikt)"("Maximum"=w247) -> ()  [unwired: 2 in, 2 out]
            n307 = property on="gehe zur zeile" class="DigWert (strikt)"("Maximum"=w247) -> ()  [unwired: 2 in, 2 out]
            n308 = property on="Einzeiln" class="Bool. (strikt)"("Disabled"=w245) -> ()  [unwired: 2 in, 2 out]
            n309 = property on="Realtime?" class="Bool. (strikt)"("Disabled"=w245) -> ()  [unwired: 2 in, 2 out]
            n310 = property on="Play" class="Bool. (strikt)"("Disabled"=w245) -> ()  [unwired: 2 in, 2 out]
          }
          frame True {
            n311 = case shown="FALSE" "min.Sound" {
              selector: "min.Sound" -> [w260 _]
              tunnel: [w260 w261] -> w254
              frame False {
              }
              frame True {
                n312 = local read "Volume"() -> (w262:i64)
                n313 = Less Or Equal?(x=w262, y=i64 10) -> (x <= y?=w261:bool)
                n314 = case shown="TRUE" w261 {
                  frame False {
                  }
                  frame True {
                    n315 = invoke on="Volume" class="Schieberegler (strikt)" method="ObjMarkieren"() -> ()  [unwired: 3 in, 3 out]
                  }
                }
              }
            }
            n316 = case shown="FALSE" "max.Sound" {
              selector: "max.Sound" -> [w256 _]
              tunnel: [w256 w257] -> w250
              frame False {
              }
              frame True {
                n317 = local read "Volume"() -> (w259:i64)
                n318 = Greater Or Equal?(x=w259, y=80) -> (x >= y?=w257:bool)
                n319 = case shown="TRUE" w257 {
                  frame False {
                  }
                  frame True {
                    n320 = invoke on="Volume" class="Schieberegler (strikt)" method="ObjMarkieren"() -> ()  [unwired: 3 in, 3 out]
                  }
                }
              }
            }
            n321 = Not(x=w254) -> (.not. x?=w252:bool)
            n322 = Not(x=w250) -> (.not. x?=w251:bool)
            n323 = And(x=w252, y=w251) -> (x .and. y?=w249:bool)
            n324 = case shown="TRUE" w249 {
              frame False {
                w264 = FALSE
                n325 = local write "Play?"(w264) -> ()
                n326 = local write "Play"(w264) -> ()
                n327 = local write "Einzeiln"(w264) -> ()
                n328 = local write "Einzeiln 2"(w264) -> ()
                n329 = local write "nach diesem lied stoppen"(w264) -> ()
              }
              frame True {
                n330 = stacked-sequence {
                  frame #0 {
                    n331 = local read "Einzeiln 2"() -> (w267:bool)
                    n332 = local write "Gespielte Lieder tabelle"(string[][] [] ("Gespielte Lieder")) -> ()
                    n333 = while {
                      shift-right: [w272] -> _
                      shift-left: 0 -> [w271]
                      stop <- w268 stop-if-true
                      n334 = local read "Playlist"() -> (w276:string[][])
                      n335 = Wait Until Next ms Multiple(millisecond multiple=50) -> ()  [unwired: 1 out]
                      n336 = Index Array(array=w276, index (row)=w271, index (col)=0) -> (element=w274:string)
                      n337 = Equal?(x=w274, y="") -> (x = y?=w268:bool)
                      n338 = case shown="FALSE" w268 {
                        tunnel: [w279 w280] -> w272
                        tunnel: w271 -> [w278 w280]
                        tunnel: [w277 w280] -> w270
                        frame False {
                          n339 = local read "Lieder:"() -> (w277:dbl)
                          n340 = Increment(x=w278) -> (x+1=w279:i32)
                        }
                        frame True {
                        }
                      }
                      "Lieder:" <- w270
                    }
                    n341 = case shown="FALSE" w267 {
                      frame False {
                      }
                      frame True {
                        n342 = local read "Pfad"() -> (w285:path)
                        n343 = call <vilib>:"Check if File or Folder Exists.vi"("path"=w285) -> ("file or folder exists?"=w287:bool)  [unwired: 1 in, 9 out]
                        n344 = call <vilib>:"Get File Extension.vi"("file"=w285) -> ("lowercase file extension"=w284:string)  [unwired: 1 in, 9 out]
                        n345 = Not(x=w287) -> (.not. x?=w286:bool)
                        n346 = Equal?(x=w284, y="wav") -> (x = y?=w282:bool)
                        n347 = call "Meldung an Benutzer5"("Enable"=w286) -> ()  [unwired: 2 in, 9 out]
                        n348 = Not(x=w282) -> (.not. x?=w281:bool)
                        n349 = call "Meldung an Benutzer6"("Enable"=w281) -> ()  [unwired: 2 in, 9 out]
                      }
                    }
                  }
                  frame #1 {
                    w288 = 1
                    # "2147483647"
                    n350 = local read "Lieder:"() -> (w289:dbl)
                    n351 = stacked-sequence {
                      frame #0 {
                        w593 = FALSE
                        n352 = local write "Stop"(FALSE) -> ()
                        n353 = local write "Start?"(TRUE) -> ()
                        n354 = local write "Play"(w593) -> ()
                        n355 = local write "Einzeiln"(w593) -> ()
                      }
                    }
                    n356 = while {
                      stop <- w331 stop-if-true
                      n357 = Wait Until Next ms Multiple(millisecond multiple=50) -> ()  [unwired: 1 out]
                      n358 = local write "nächtes lied"(FALSE) -> ()
                      n359 = case shown="TRUE" "nächtes lied" {
                        frame False {
                        }
                        frame True {
                          n360 = stacked-sequence {
                            frame #0 {
                            }
                          }
                        }
                      }
                      n361 = case shown="TRUE" "nächtes lied" {
                        frame False {
                        }
                        frame True {
                          n362 = stacked-sequence {
                            frame #0 {
                              n363 = local write "Seite"(0) -> ()
                              n364 = local write "end of file?"(TRUE) -> ()
                              n365 = property on="nächtes lied" class="Bool. (strikt)"("Disabled"=2) -> ()  [unwired: 2 in, 2 out]
                            }
                            frame #1 {
                              n366 = call "Verzögerung3"() -> ()  [unwired: 2 in, 10 out]
                            }
                            frame #2 {
                              n367 = property on="nächtes lied" class="Bool. (strikt)"("Disabled"=0) -> ()  [unwired: 2 in, 2 out]
                            }
                          }
                        }
                      }
                      n368 = local write "go to line?"("gehe zur zeile kn.") -> ()
                      n369 = case shown="TRUE" "gehe zur zeile kn." {
                        frame False {
                        }
                        frame True {
                          n370 = stacked-sequence {
                            frame #0 {
                              w332 = 2
                              n371 = local write "Seite"(0) -> ()
                              n372 = local write "end of file?"(TRUE) -> ()
                              n373 = property on="gehe zur zeile" class="DigWert (strikt)"("Disabled"=w332) -> ()  [unwired: 2 in, 2 out]
                              n374 = property on="gehe zur zeile kn." class="Bool."("Disabled"=w332) -> ()  [unwired: 2 in, 2 out]
                            }
                            frame #1 {
                              n375 = while {
                                stop <- w338 stop-if-true
                                n376 = Wait Until Next ms Multiple(millisecond multiple=50) -> ()  [unwired: 1 out]
                                n377 = local read "gehe zur zeile"() -> (w335:dbl)
                                n378 = local read "Spalte"() -> (w337:dbl)
                                n379 = Decrement(x=w335) -> (x-1=w336:dbl)
                                n380 = Equal?(x=w337, y=w336) -> (x = y?=w338:bool)
                              }
                            }
                            frame #2 {
                              w340 = 0
                              n381 = property on="gehe zur zeile kn." class="Bool."("Disabled"=w340) -> ()  [unwired: 2 in, 2 out]
                              n382 = property on="gehe zur zeile" class="DigWert (strikt)"("Disabled"=w340) -> ()  [unwired: 2 in, 2 out]
                            }
                          }
                        }
                      }
                      n383 = local read "Stop?"() -> (w331:bool)
                    }
                    n384 = call <vilib>:"Intialize Keyboard.vi"() -> ("error out"=w292:errorcluster, "device ID"=w294:refnum<k1>)  [unwired: 1 in, 9 out]
                    n385 = while {
                      stop <- w347 stop-if-true
                      n386 = Wait Until Next ms Multiple(millisecond multiple=50) -> ()  [unwired: 1 out]
                      n387 = case shown="0, Voreinstellung" "Seite" {
                        frame 0, Default {
                          n388 = local read "Einzeiln 2"() -> (w348:bool)
                          n389 = case shown="FALSE" w348 {
                            tunnel: [w371 w497] -> w349
                            frame False {
                              # "allle true = true sonst false"
                              n390 = local read "end of file?"() -> (w368:bool)
                              n391 = local read "Spalte"() -> (w374:dbl)
                              n392 = case shown="FALSE" "von, bis" {
                                tunnel: w374 -> [w441 w453]
                                tunnel: w368 -> [w440 _]
                                tunnel: [w439 w452] -> w364
                                frame False {
                                n393 = case shown="TRUE" w440 {
                                tunnel: w441 -> [w442 w445]
                                tunnel: [w442 w444] -> w439
                                frame False {
                                }
                                frame True {
                                n394 = case shown="FALSE" "go to line?" {
                                tunnel: w445 -> [w448 _]
                                tunnel: [w447 w449] -> w444
                                frame False {
                                n395 = local write "end of file?"(FALSE) -> ()
                                n396 = Increment(x=w448) -> (x+1=w447:dbl)
                                }
                                frame True {
                                n397 = Decrement(x="gehe zur zeile") -> (x-1=w449:dbl)
                                }
                                }
                                }
                                }
                                }
                                frame True {
                                n398 = local read "nächtes lied"() -> (w451:bool)
                                n399 = case shown="FALSE" w451 {
                                tunnel: w453 -> [w456 w489]
                                tunnel: [w460 w490] -> w452
                                frame False {
                                n400 = flat-sequence {
                                tunnel: [w468] -> w461
                                tunnel: w456 -> [w467]
                                tunnel: [w466] -> w457
                                tunnel: w456 -> [w466]
                                tunnel: [w463] -> w455
                                tunnel: [w462] -> w454
                                tunnel: w461 -> [w473]
                                tunnel: [w474] -> w459
                                tunnel: [w472] -> w458
                                tunnel: w457 -> [w472]
                                tunnel: w455 -> [w471]
                                tunnel: w454 -> [w470]
                                tunnel: [w488] -> w460
                                tunnel: w459 -> [w488]
                                tunnel: w458 -> [_]
                                frame #0 {
                                n401 = Decrement(x="from") -> (x-1=w463:dbl)
                                n402 = Increment(x=w467) -> (x+1=w468:dbl)
                                n403 = Decrement(x="to") -> (x-1=w462:dbl)
                                }
                                frame #1 {
                                n404 = case shown="TRUE" "Start?" {
                                tunnel: [w478 w486] -> w474
                                tunnel: w473 -> [w477 _]
                                tunnel: w471 -> [w476 w486]
                                tunnel: w470 -> [w475 _]
                                frame False {
                                n405 = Less? "Kleiner?"(x=w477, y=w476) -> (x < y?=w479:bool)
                                n406 = Greater? "Größer?"(x=w477, y=w475) -> (0:w480:bool)
                                n407 = case shown="FALSE" w479 {
                                tunnel: [w484 w485] -> w481
                                tunnel: w477 -> [w484 _]
                                tunnel: w476 -> [_ w485]
                                frame False {
                                }
                                frame True {
                                }
                                }
                                n408 = case shown="TRUE" w480 {
                                tunnel: w481 -> [w482 _]
                                tunnel: [w482 w483] -> w478
                                tunnel: w476 -> [_ w483]
                                frame False {
                                }
                                frame True {
                                }
                                }
                                }
                                frame True {
                                n409 = stacked-sequence {
                                frame #0 {
                                n410 = local write "Start?"(FALSE) -> ()
                                }
                                }
                                }
                                }
                                }
                                frame #2 {
                                }
                                }
                                }
                                frame True {
                                n411 = Increment(x=w489) -> (x+1=w490:dbl)
                                }
                                }
                                }
                              }
                              n412 = local read "nächtes lied"() -> (w360:bool)
                              n413 = local read "go to line?"() -> (w361:bool)
                              n414 = Or(x=w361, y=w360) -> (x .or. y?=w359:bool)
                              n415 = Not(x=w359) -> (.not. x?=w358:bool)
                              n416 = And(x="zufall", y=w358) -> (x .and. y?=w362:bool)
                              n417 = case shown="FALSE" w362 {
                                tunnel: w364 -> [w377 w380]
                                tunnel: [w377 w379] -> w363
                                frame False {
                                }
                                frame True {
                                n418 = while {
                                tunnel: w380 -> [w385]
                                tunnel: [w391] -> w379
                                shift-right: [w387] -> _
                                shift-left: 0 -> [w386]
                                stop <- w392 stop-if-true
                                n419 = local read "gespielte Lieder:"() -> (w389:dbl)
                                n420 = Wait Until Next ms Multiple(millisecond multiple=50) -> ()  [unwired: 1 out]
                                n421 = Not(x="Wiederholen?") -> (.not. x?=w384:bool)
                                n422 = Equal?(x=w389, y="zu spielende Lieder:") -> (x = y?=w382:bool)
                                n423 = And(x=w384, y=w382) -> (x .and. y?=w383:bool)
                                n424 = case shown="TRUE" "Wiederholen?" {
                                tunnel: w382 -> [_ w394]
                                frame False {
                                }
                                frame True {
                                n425 = case shown="TRUE" w394 {
                                frame False {
                                }
                                frame True {
                                n426 = local write "Gespielte Lieder tabelle"(string[][] [] ("Gespielte Lieder tabelle")) -> ()
                                }
                                }
                                }
                                }
                                n427 = case shown="FALSE" w383 {
                                tunnel: [w399 TRUE] -> w392
                                tunnel: [w396 w429] -> w390
                                tunnel: w386 -> [w398 _]
                                tunnel: [w397 0] -> w387
                                frame False {
                                n428 = case shown="1.." w398 {
                                tunnel: [FALSE w419] -> w399
                                selector: w398 -> [w401 w417]
                                tunnel: [w402 w418] -> w397
                                tunnel: [0 ("uniform (discrete) random data[0]") w416] -> w396
                                frame ..0 {
                                n429 = local read "von, bis"() -> (w410:bool)
                                n430 = Increment(x=w401) -> (x+1=w402:i32)
                                n431 = case shown="TRUE" w410 {
                                tunnel: [0 w414] -> w405
                                tunnel: [w411 w415] -> w409
                                frame False {
                                n432 = local read "Lieder:"() -> (w412:dbl)
                                n433 = Decrement(x=w412) -> (x-1=w411:dbl)
                                }
                                frame True {
                                n434 = local read "from"() -> (w414:dbl)
                                n435 = local read "to"() -> (w415:dbl)
                                }
                                }
                                n436 = call-poly <vilib>:"Discrete Random.vi"("seed"=w405, "reset"=FALSE, "n"=w409, "samples"=1) -> ("uniform (discrete) random data"=w407:i32[])  [unwired: 7 out]
                                n437 = Array To Cluster(array=w407) -> (cluster=→"Cluster":T1)
                                }
                                frame 1.. {
                                n438 = local read "Gespielte Lieder tabelle"() -> (w421:string[][])
                                n439 = local read "Cluster"() -> (w420:T1)
                                n440 = Unbundle(w420) -> ("uniform (discrete) random data[0]"=w416:i32)  [unwired: 8 out]
                                n441 = Index Array(array=w421, index (row)=w416, index (col)=0 ("Deaktivierter Index (Spalte)")) -> (element=w423:string)
                                n442 = Equal?(x=w423, y="") -> (x = y?=w419:bool)
                                n443 = case shown="FALSE" w419 {
                                tunnel: [0 w426] -> w418
                                tunnel: w417 -> [_ w426]
                                frame False {
                                }
                                frame True {
                                }
                                }
                                }
                                }
                                }
                                frame True {
                                n444 = local read "Lieder:"() -> (w429:dbl)
                                }
                                }
                                n445 = case shown="TRUE" w392 {
                                tunnel: w385 -> [w430 _]
                                tunnel: [w430 w431] -> w391
                                tunnel: w390 -> [_ w431]
                                frame False {
                                }
                                frame True {
                                }
                                }
                                }
                                }
                              }
                              n446 = local read "Wiederholen?"() -> (w351:bool)
                              n447 = local read "Lerrerpad?"() -> (w366:bool)
                              n448 = Compound Arithmetic op=OR("von, bis", w351) -> (w353:bool)
                              n449 = case shown="TRUE" w351 {
                                tunnel: w366 -> [_ w435]
                                tunnel: w363 -> [w432 w434]
                                tunnel: [w432 w433] -> w356
                                frame False {
                                }
                                frame True {
                                n450 = case shown="TRUE" w435 {
                                tunnel: w434 -> [w436 _]
                                tunnel: [w436 0] -> w433
                                frame False {
                                }
                                frame True {
                                }
                                }
                                }
                              }
                              n451 = case shown="FALSE" "nach diesem lied stoppen" {
                                tunnel: [w375 w376] -> w357
                                tunnel: w356 -> [w375 _]
                                frame False {
                                }
                                frame True {
                                n452 = local read "Lieder:"() -> (w376:dbl)
                                }
                              }
                              "Spalte" <- w357
                              n453 = Index Array(array="Playlist", index (row)=w357, index (col)=0) -> (element=w371:string)
                              n454 = local read "Seite"() -> (w367:dbl)
                              n455 = Equal?(x=w371, y="") -> (x = y?=w354:bool)
                              "Lerrerpad?" <- w354
                              n456 = Or(x="nach diesem lied stoppen", y=w354) -> (x .or. y?=w355:bool)
                              n457 = case shown="TRUE" w354 {
                                tunnel: w367 -> [_ w492]
                                tunnel: [1 w492] -> w373
                                frame False {
                                }
                                frame True {
                                }
                              }
                              n458 = case shown="TRUE" w353 {
                                tunnel: w355 -> [w438 _]
                                frame False {
                                n459 = local write "Stop?"(w438) -> ()
                                }
                                frame True {
                                }
                              }
                              n460 = local write "Seite"(w373) -> ()
                            }
                            frame True {
                              n461 = local read "Wiederholen?"() -> (w494:bool)
                              n462 = local read "end of file?"() -> (w495:bool)
                              n463 = case shown="TRUE" w495 {
                                tunnel: w494 -> [_ w501]
                                tunnel: [FALSE w500] -> w493
                                frame False {
                                n464 = local write "Seite"(1) -> ()
                                }
                                frame True {
                                n465 = case shown="TRUE" w501 {
                                tunnel: [TRUE FALSE] -> w500
                                frame False {
                                }
                                frame True {
                                n466 = local write "Seite"(1) -> ()
                                }
                                }
                                }
                              }
                              n467 = local write "Stop?"(w493) -> ()
                              n468 = Path To String(path="Pfad") -> (string=w497:string)
                            }
                          }
                          "Gelesener Pfad" <- w349
                        }
                        frame 1 {
                          (unwired) 0
                          w517 = T6 1 items=["Endliche Anzahl", "Kontinuierlich"] ("sample mode")
                          n469 = local read "Gelesener Pfad"() -> (w513:string)
                          n470 = String To Path(string=w513) -> (path=w514:path)
                          n471 = case shown="FALSE" "Realtime?" {
                            tunnel: [100000 10000] -> w516
                            frame False {
                            }
                            frame True {
                            }
                          }
                          n472 = local read "Spalte"() -> (w509:dbl)
                          n473 = Increment(x="gespielte Lieder:") -> (x+1=w505:dbl)
                          n474 = Initialize Array("gespielt", 1 ("Dimension")) -> (w510:string[])
                          n475 = local write "gespielte Lieder:"(w505) -> ()
                          n476 = Insert Into Array(array="Gespielte Lieder tabelle", index (row)=w509, new element=w510) -> (w507:string[][])  [unwired: 1 in]
                          n477 = call-poly <vilib>:"Sound File Info.vi"("path"=w514) -> ("error out"=w525:errorcluster, "sound format"=w532:T7, "path out"=w518:path)  [unwired: 1 in, 7 out]
                          n478 = local write "Gespielte Lieder tabelle"(w507) -> ()
                          n479 = call-poly <vilib>:"Sound File Open.vi"("error in (no error)"=w525, "path"=w518) -> ("error out"=w524:errorcluster, "sound file refnum"=w519:T8)  [unwired: 8 out]
                          n480 = call <vilib>:"Sound Output Configure.vi"("number of samples/ch"=w516, "sample mode"=w517, "error in (no error)"=w524, "sound format"=w532, "device ID"="device ID") -> ("error out"=w530:errorcluster, "task ID"=w529:T9)  [unwired: 5 out]
                          n481 = while {
                            shift-right: [w552] -> w528
                            shift-left: w529 -> [w553]
                            shift-right: [w547] -> w526
                            shift-left: w519 -> [w554]
                            shift-right: [w535] -> w527
                            shift-left: w530 -> [w548]
                            tunnel: [2] -> _
                            stop <- w545 stop-if-true
                            w549 = T10 2 items=["Absolut"=0, "Relativ"=2] ("position mode")
                            w536 = 2
                            n482 = local read "Pause"() -> (w542:bool)
                            n483 = case shown="TRUE" w542 {
                              frame False {
                              }
                              frame True {
                                n484 = Wait Until Next ms Multiple(millisecond multiple=50) -> ()  [unwired: 1 out]
                              }
                            }
                            n485 = property on="Einzeiln" class="Bool. (strikt)"("Disabled"=w536) -> (error out=w541:errorcluster)  [unwired: 2 in, 1 out]
                            n486 = case shown="FALSE" "Pause" {
                              tunnel: w554 -> [w571 w583]
                              tunnel: w553 -> [w568 w584]
                              tunnel: [w567 w584] -> w552
                              tunnel: [w566 w582] -> w535
                              tunnel: 100000 -> [w565 _]
                              tunnel: w549 -> [w564 _]
                              tunnel: w548 -> [w563 w582]
                              tunnel: [w562 w583] -> w547
                              frame False {
                                n487 = call-poly <vilib>:"Sound File Read.vi"("number of samples/ch (-1: all)"=w565, "error in (no error)"=w563, "position mode"=w564, "sound file refnum"=w571) -> ("error out"=w570:errorcluster, "data"=w569:waveform(dbl)[], "sound file refnum out"=w562:T8, "end of file?"=→"end of file?":bool)  [unwired: 1 in, 3 out]
                                n488 = local read "background"() -> (w560:bool)
                                n489 = case shown="FALSE" w560 {
                                tunnel: [w572 50] -> w559
                                tunnel: "Volume" -> [w572 _]
                                frame False {
                                }
                                frame True {
                                }
                                }
                                n490 = stacked-sequence {
                                tunnel: w559 -> [w581]
                                tunnel: w570 -> [w580]
                                tunnel: w569 -> [w578]
                                tunnel: w568 -> [w577]
                                tunnel: [w575] -> w567
                                tunnel: [w574] -> w566
                                frame #0 {
                                n491 = call-poly <vilib>:"Sound Output Set Volume.vi"("error in (no error)"=w580, "volume"=w581, "task ID"=w577) -> ("error out"=w579:errorcluster, "task ID out"=w576:T9)  [unwired: 7 out]
                                n492 = call-poly <vilib>:"Sound Output Write.vi"("error in (no error)"=w579, "data"=w578, "task ID"=w576) -> ("error out"=w574:errorcluster, "task ID out"=w575:T9)  [unwired: 1 in, 6 out]
                                }
                                }
                              }
                              frame True {
                              }
                            }
                            n493 = property on="Play" class="Bool. (strikt)"(error in=w541, "Disabled"=w536) -> (error out=w537:errorcluster)  [unwired: 1 in, 1 out]
                            n494 = property on="Realtime?" class="Bool. (strikt)"(error in=w537, "Disabled"=w536) -> ()  [unwired: 1 in, 2 out]
                            n495 = stacked-sequence {
                              tunnel: [w590] -> w545
                              tunnel: w535 -> [w591]
                              tunnel: [w589] -> w539
                              tunnel: [w586] -> w538
                              frame #0 {
                                n496 = Unbundle By Name(w591) -> ("status"=w589:bool)
                                n497 = local read "Stop?"() -> (w585:bool)
                                n498 = local read "end of file?"() -> (w588:bool)
                                n499 = Or(x="Stop", y=w585) -> (x .or. y?=w586:bool)
                                n500 = Compound Arithmetic op=OR(w589, w586, w588) -> (w590:bool)
                              }
                            }
                            n501 = local read "Seite"() -> (w543:dbl)
                            n502 = Or(x=w539, y=w538) -> (x .or. y?=→"Stop?":bool)
                            n503 = case shown="TRUE" w545 {
                              tunnel: [w556 0] -> w544
                              tunnel: w543 -> [w556 _]
                              frame False {
                              }
                              frame True {
                              }
                            }
                            n504 = local write "Seite"(w544) -> ()
                          }
                          n505 = call <vilib>:"Sound File Close.vi"("error in (no error)"=w527, "sound file refnum"=w526) -> ("error out"=w520:errorcluster)  [unwired: 9 out]
                          n506 = call <vilib>:"Sound Output Wait.vi"("error in (no error)"=w520, "task ID"=w528) -> ("error out"=w522:errorcluster, "task ID out"=w523:T9)  [unwired: 1 in, 7 out]
                          n507 = call <vilib>:"Sound Output Clear.vi"("error in (no error)"=w522, "task ID"=w523) -> ("error out"=w521:errorcluster)  [unwired: 9 out]
                          n508 = call <vilib>:"Simple Error Handler.vi"("error in (no error)"=w521) -> ()  [unwired: 1 in, 8 out]
                        }
                      }
                      n509 = local read "Stop?"() -> (w347:bool)
                    }
                    n510 = while {
                      shift-right: [w296] -> _
                      shift-left: 0 -> [w295]
                      stop <- w298 stop-if-true
                      n511 = Wait Until Next ms Multiple(millisecond multiple=50) -> ()  [unwired: 1 out]
                      n512 = case shown="TRUE" "counter" {
                        tunnel: w295 -> [w300 w304]
                        tunnel: [w300 w305] -> w296
                        frame False {
                        }
                        frame True {
                          n513 = flat-sequence {
                            tunnel: w304 -> [_]
                            tunnel: [w308] -> w303
                            tunnel: [w307] -> w302
                            tunnel: [w306] -> w301
                            tunnel: [w310] -> w305
                            tunnel: w303 -> [w312]
                            tunnel: w302 -> [w311]
                            tunnel: w301 -> [w309]
                            frame #0 {
                              n514 = local read "Volume"() -> (w306:i64)
                              n515 = call "Counter.vi"() -> ("Way 2"=w307:enum32{"Up", "Down"}, "End 2"=w308:dbl)  [unwired: 1 in, 9 out]
                            }
                            frame #1 {
                              n516 = while {
                                tunnel: w312 -> [w322]
                                tunnel: w311 -> [w321]
                                shift-right: [w320] -> w310
                                shift-left: w309 -> [w319]
                                i -> [w315]
                                stop <- w314 stop-if-true
                                n517 = local write "Volume"(w319) -> ()
                                n518 = case shown="\"Up\", Voreinstellung" w321 {
                                tunnel: [w324 w326] -> w320
                                tunnel: w319 -> [w323 w325]
                                frame "Up", Default {
                                n519 = Increment(x=w323) -> (x+1=w324:i64)
                                }
                                frame "Down" {
                                n520 = Decrement(x=w325) -> (x-1=w326:i64)
                                }
                                }
                                n521 = Equal?(x=w319, y=w322) -> (x = y?=w318:bool)
                                n522 = Equal?(x=101, y=w315) -> (x = y?=w313:bool)
                                n523 = Wait Until Next ms Multiple(millisecond multiple=50) -> ()  [unwired: 1 out]
                                n524 = Or(x=w318, y=w313) -> (x .or. y?=w314:bool)
                              }
                            }
                          }
                        }
                      }
                      n525 = local read "Stop?"() -> (w298:bool)
                    }
                    n526 = while {
                      tunnel: w294 -> [w618]
                      tunnel: [w615] -> w293
                      tunnel: w292 -> [w616]
                      shift-right: [w607] -> _
                      shift-left: 0 -> [w606]
                      stop <- w612 stop-if-true
                      n527 = local read "Stop"() -> (w611:bool)
                      n528 = call-poly <vilib>:"Acquire Input Data.vi"("device ID"=w618, "error in (no error)"=w616) -> ("device ID"=w615:refnum<k1>, "keys pressed"=w614:T11)  [unwired: 16 out]
                      n529 = Wait Until Next ms Multiple(millisecond multiple=50) -> ()  [unwired: 1 out]
                      n530 = case shown="TRUE" w611 {
                        frame False {
                        }
                        frame True {
                          w671 = FALSE
                          n531 = local write "Wiederholen?"(w671) -> ()
                          n532 = local write "Wiederholen"(w671) -> ()
                          n533 = local write "Einzeiln 2"(w671) -> ()
                        }
                      }
                      n534 = Array To Cluster(array=w614) -> (cluster=w613:T12)
                      n535 = Or(x=T4."RCONTROL" ("keyType 3"), y=T4."LCONTROL" ("keyType 3")) -> (x .or. y?=w610:i32)
                      n536 = Unbundle(w613) -> ("keys pressed[0]"=w603:T4, "keys pressed[1]"=w602:T4, "keys pressed[2]"=w601:T4, "keys pressed[3]"=w600:T4, "keys pressed[4]"=w599:T4, "keys pressed[5]"=w598:T4, "keys pressed[6]"=w597:T4, "keys pressed[7]"=w596:T4, "keys pressed[8]"=w595:T4)
                      n537 = Equal?(x=w603, y=w610) -> ()  [unwired: 1 out]
                      n538 = case shown="TRUE" "shortcut's" {
                        tunnel: w603 -> [_ w642]
                        tunnel: w602 -> [_ w641]
                        tunnel: w601 -> [_ w640]
                        tunnel: w600 -> [_ w639]
                        tunnel: w599 -> [_ w638]
                        tunnel: w598 -> [_ w637]
                        tunnel: w597 -> [_ w636]
                        tunnel: w596 -> [_ w635]
                        tunnel: w595 -> [_ w634]
                        frame False {
                        }
                        frame True {
                          n539 = Compound Arithmetic op=OR(w642, w641, w640, w639, w638, w637, w636, w635, w634) -> (w643:i32)
                          n540 = Equal?(x=w643, y=T4."S" ("keyType 3")) -> (x = y?=w633:bool)
                          n541 = Equal?(x=w643, y=T4."P" ("keyType 3")) -> (x = y?=w653:bool)
                          n542 = local read "Wiederholen"() -> (w645:bool)
                          n543 = Equal?(x=w643, y=T4."B" ("keyType 3")) -> (x = y?=w650:bool)
                          n544 = Equal?(x=w643, y=T4."W" ("keyType 3")) -> (x = y?=w646:bool)
                          n545 = local read "Pause"() -> (w652:bool)
                          n546 = local read "Stop"() -> (w648:bool)
                          n547 = case shown="TRUE" w633 {
                            tunnel: w648 -> [_ w659]
                            frame False {
                            }
                            frame True {
                              n548 = stacked-sequence {
                                tunnel: w659 -> [_ _]
                                frame #0 {
                                n549 = local write "Stop"(TRUE) -> ()
                                }
                                frame #1 {
                                n550 = call "Verzögerung8"() -> ()  [unwired: 2 in, 10 out]
                                }
                              }
                            }
                          }
                          n551 = case shown="TRUE" w653 {
                            tunnel: w652 -> [_ w666]
                            frame False {
                            }
                            frame True {
                              n552 = stacked-sequence {
                                tunnel: w666 -> [w668 _]
                                frame #0 {
                                n553 = case shown="TRUE" w668 {
                                tunnel: [TRUE FALSE] -> w667
                                frame False {
                                }
                                frame True {
                                }
                                }
                                n554 = local write "Pause"(w667) -> ()
                                }
                                frame #1 {
                                n555 = call "Verzögerung"() -> ()  [unwired: 2 in, 10 out]
                                }
                              }
                            }
                          }
                          n556 = case shown="TRUE" w646 {
                            tunnel: w645 -> [_ w654]
                            frame False {
                            }
                            frame True {
                              n557 = stacked-sequence {
                                tunnel: w654 -> [w656 _]
                                frame #0 {
                                n558 = case shown="TRUE" w656 {
                                tunnel: [TRUE FALSE] -> w655
                                frame False {
                                }
                                frame True {
                                }
                                }
                                n559 = local write "Wiederholen"(w655) -> ()
                                }
                                frame #1 {
                                n560 = call "Verzögerung2"() -> ()  [unwired: 2 in, 10 out]
                                }
                              }
                            }
                          }
                          n561 = case shown="TRUE" w650 {
                            tunnel: "background" -> [_ w661]
                            frame False {
                            }
                            frame True {
                              n562 = stacked-sequence {
                                tunnel: w661 -> [w663 _]
                                frame #0 {
                                n563 = case shown="FALSE" w663 {
                                tunnel: [TRUE FALSE] -> w662
                                frame False {
                                }
                                frame True {
                                }
                                }
                                n564 = local write "background"(w662) -> ()
                                }
                                frame #1 {
                                n565 = call "Verzögerung7"() -> ()  [unwired: 2 in, 10 out]
                                }
                              }
                            }
                          }
                        }
                      }
                      n566 = case shown="TRUE" FALSE {
                        tunnel: w606 -> [w619 w623]
                        tunnel: [w619 w622] -> w607
                        tunnel: [FALSE w621] -> _
                        frame False {
                        }
                        frame True {
                          n567 = case shown="0, Voreinstellung" w623 {
                            selector: w623 -> [w624 w628 _]
                            tunnel: [w625 w629 0] -> w622
                            tunnel: [TRUE TRUE FALSE] -> w621
                            frame 0, Default {
                              n568 = Increment(x=w624) -> (x+1=w625:i32)
                            }
                            frame 1 {
                              n569 = call "Verzögerung9"() -> ()  [unwired: 2 in, 10 out]
                              n570 = Increment(x=w628) -> (x+1=w629:i32)
                            }
                            frame 2 {
                            }
                          }
                        }
                      }
                      n571 = local read "Stop?"() -> (w612:bool)
                    }
                    n572 = property on="from" class="DigWert (strikt)"("Maximum"=w289, "Minimum"=w288) -> ()  [unwired: 2 in, 2 out]
                    n573 = property on="to" class="DigWert (strikt)"("Maximum"=w289, "Minimum"=w288) -> ()  [unwired: 2 in, 2 out]
                    n574 = property on="gehe zur zeile" class="DigWert (strikt)"("Maximum"=w289, "Minimum"=w288) -> ()  [unwired: 2 in, 2 out]
                    n575 = call-poly <vilib>:"Close Input Device.vi"("device ID"=w293) -> ()  [unwired: 1 in, 9 out]
                  }
                }
              }
            }
          }
        }
      }
      n576 = while {
        tunnel: w225 -> [w774]
        stop <- FALSE stop-if-true
        (unwired) 0
        n577 = event shown="[8] \"liste löschen\": Wertänderung" {
          selector: _ -> [_ _ _ _ _ _ _ _ _ _ _ _ _ _ _]
          dyn-events: _ -> [_ _ _ _ _ _ _ _ _ _ _ _ _ _ _]
          timeout: _ -> [_ _ _ _ _ _ _ _ _ _ _ _ _ _ _]
          tunnel: w774 -> [_ _ _ _ w869 _ _ _ _ _ _ _ _ _ _]
          event "Hinzufügen": Value Change {
            w777 = 0
            n578 = event-data() -> ("NewVal"=w779:bool)  [unwired: 6 out]
            n579 = local read "Pfad"() -> (w781:path)
            n580 = call <vilib>:"Get File Extension.vi"("file"=w781) -> ("filename without extension"=w778:string, "lowercase file extension"=w780:string)  [unwired: 1 in, 8 out]
            n581 = while {
              tunnel: w781 -> [w791]
              tunnel: w780 -> [w790]
              tunnel: w779 -> [w788]
              tunnel: w778 -> [w783]
              shift-right: [w785] -> _
              shift-left: w777 -> [w784]
              shift-right: [w786] -> _
              shift-left: w777 -> [w787]
              stop <- w782 stop-if-true
              n582 = Equal?(x=w790, y="wav") -> (x = y?=w792:bool)
              n583 = case shown="TRUE" w788 {
                tunnel: w791 -> [_ w803]
                tunnel: w792 -> [_ w802]
                tunnel: [w795 w801] -> w786
                tunnel: w787 -> [w795 w800]
                tunnel: [w794 w799] -> w785
                tunnel: w784 -> [w794 w798]
                tunnel: w783 -> [_ w797]
                tunnel: [TRUE w796] -> w782
                frame False {
                }
                frame True {
                  n584 = case shown="TRUE" w802 {
                    tunnel: w803 -> [_ w813]
                    tunnel: [w806 w812] -> w801
                    tunnel: w800 -> [w806 w811]
                    tunnel: w798 -> [w805 w810]
                    tunnel: [w805 w809] -> w799
                    tunnel: w797 -> [_ w808]
                    tunnel: [TRUE w807] -> w796
                    frame False {
                      n585 = call "Meldung an Benutzer2"() -> ()  [unwired: 3 in, 9 out]
                    }
                    frame True {
                      n586 = case shown="1" w811 {
                        selector: w811 -> [w814 w833]
                        tunnel: w813 -> [_ w834]
                        tunnel: [w817 w833] -> w812
                        tunnel: w810 -> [w818 w832]
                        tunnel: [w819 w832] -> w809
                        tunnel: w808 -> [_ w831]
                        tunnel: [FALSE w830] -> w807
                        frame 0, Default {
                          n587 = local read "Playlist"() -> (w823:string[][])
                          n588 = Index Array(array=w823, index (row)=w818, index (col)=0 ("Deaktivierter Index (Spalte)")) -> (element=w821:string)
                          n589 = Equal?(x=w821, y="") -> (x = y?=w816:bool)
                          n590 = case shown="TRUE" w816 {
                            tunnel: [w825 w827] -> w819
                            tunnel: w818 -> [w824 w827]
                            tunnel: w814 -> [w826 w829]
                            tunnel: [w826 w828] -> w817
                            frame False {
                              n591 = Increment(x=w824) -> (x+1=w825:i32)
                            }
                            frame True {
                              n592 = Increment(x=w829) -> (x+1=w828:i32)
                            }
                          }
                        }
                        frame 1 {
                          n593 = stacked-sequence {
                            tunnel: w834 -> [w841 _]
                            tunnel: w832 -> [w838 _]
                            tunnel: w831 -> [w837 _]
                            tunnel: [_ TRUE] -> w830
                            frame #0 {
                              n594 = property on="Playlist 2" class="Listenfeld (strikt)"() -> ("Item Names"=w836:string[])  [unwired: 2 in, 2 out]
                              n595 = Path To String(path=w841) -> (string=w843:string)
                              n596 = Initialize Array(w837, 1) -> (w839:string[])
                              n597 = local read "Playlist"() -> (w846:string[][])
                              n598 = Insert Into Array(array=w836, index=w838, new element=w839) -> (w835:string[])
                              n599 = Initialize Array(w843, 1) -> (w844:string[])
                              n600 = property on="Playlist 2" class="Listenfeld (strikt)"("Item Names"=w835) -> ()  [unwired: 2 in, 2 out]
                              n601 = Insert Into Array(array=w846, index (row)=w838, new element=w844) -> (w842:string[][])  [unwired: 1 in]
                              n602 = local write "Playlist"(w842) -> ()
                            }
                            frame #1 {
                            }
                          }
                        }
                      }
                    }
                  }
                }
              }
            }
          }
          event "Info": Value Change {
            n603 = event-data() -> ("NewVal"=w848:bool)  [unwired: 6 out]
            n604 = case shown="TRUE" w848 {
              frame False {
              }
              frame True {
                n605 = call "Info.vi"() -> ()  [unwired: 1 out]
              }
            }
          }
          event "playlist speichern": Value Change {
            n606 = event-data() -> ("NewVal"=w849:bool)  [unwired: 6 out]
            n607 = case shown="TRUE" w849 {
              frame False {
              }
              frame True {
                n608 = Open/Create/Replace File(prompt="save Playlist" ("Eingabeaufforderung"), operation (0:open)=T2."open or create" ("Operation (0:Öffnen)"), access (0:read/write)=enum16{"read/write", "read-only", "write-only"}."read/write" ("Zugriff (0:Lesen/Schreiben)")) -> (refnum out=w855:refnum<file>, cancelled=w854:bool, error out=w853:errorcluster)  [unwired: 1 in, 2 out]
                n609 = local write "Fehler (Ausgang)"(w853) -> ()
                n610 = case shown="FALSE" w854 {
                  tunnel: w855 -> [w856 _]
                  frame False {
                    n611 = local read "Playlist"() -> (w859:string[][])
                    n612 = Refnum to Path(1:w856) -> (0:w857:path)
                    n613 = call-poly <vilib>:"Write To Spreadsheet File.vi"("append to file? (new file:F)"=FALSE, "2D data"=w859, "file path (dialog if empty)"=w857) -> ()  [unwired: 3 in, 3 out]
                  }
                  frame True {
                  }
                }
              }
            }
          }
          event "Schließen.": Value Change {
            n614 = event-data() -> ("NewVal"=w860:bool)  [unwired: 6 out]
            n615 = case shown="TRUE" w860 {
              frame False {
              }
              frame True {
                n616 = local read "Deutsch?"() -> (w862:bool)
                n617 = case shown="FALSE" w862 {
                  tunnel: [w863 w866] -> w861
                  frame False {
                    n618 = call "Meldung an Benutzer"("Message"="Do you really want to exit?") -> ("Yes"=w863:bool)  [unwired: 2 in, 8 out]
                  }
                  frame True {
                    n619 = call "Meldung an Benutzer4"("Message"="Wilst du das Programm schließen?") -> ("Ja"=w866:bool)  [unwired: 2 in, 8 out]
                  }
                }
                n620 = case shown="TRUE" w861 {
                  frame False {
                  }
                  frame True {
                    n621 = control-ref of="dieses VI"() -> (w867:refnum<vi>)
                    n622 = invoke class="\"" method="FP.Schließen"(reference=w867) -> ()  [unwired: 2 in, 3 out]
                  }
                }
              }
            }
          }
          event "Hilfe": Value Change {
            n623 = event-data() -> ()  [unwired: 7 out]
            n624 = local read "Deutsch?"() -> (w868:bool)
            n625 = case shown="FALSE" w868 {
              tunnel: ["!!!Attention!!!\nThe help is in German\nPlease choose:" ("message") "Bitte auswählen:" ("message")] -> w873
              tunnel: ["Easy" ("Left Button Text (\"Yes\")") "Einfach" ("Left Button Text (\"Yes\")")] -> w872
              tunnel: ["Exceptet" ("Center Button Text (\"No\")") "Genau" ("Center Button Text (\"No\")")] -> w871
              frame False {
              }
              frame True {
              }
            }
            n626 = call <vilib>:"Three Button Dialog.vi"("Center Button Text (\"No\")"=w871, "Left Button Text (\"Yes\")"=w872, "message"=w873) -> ("Which Button?"=w870:T13)  [unwired: 2 in, 6 out]
            n627 = case shown="\"Left Button\", Voreinstellung" w870 {
              tunnel: w869 -> [w880 _ _ _]
              frame "Left Button", Default {
                n628 = One Button Dialog(message=w880) -> ()  [unwired: 2 out]
              }
              frame "Center Button" {
              }
              frame "Right Button" {
              }
              frame "Window Close" {
              }
            }
          }
          event "Playlist": Key Down {
            n629 = event-data() -> ("VKey"=w881:T14)  [unwired: 9 out]
            n630 = while {
              shift-right: [w894] -> _
              shift-left: 0 -> [w895]
              tunnel: w881 -> [_]
              stop <- w898 stop-if-true
              n631 = local read "Playlist"() -> (w883:string[][])
              n632 = Wait Until Next ms Multiple(millisecond multiple=50) -> ()  [unwired: 1 out]
              n633 = Index Array(array=w883, index (row)=w895, index (col)=0) -> (element=w897:string)
              n634 = String To Path(string=w897) -> (path=w892:path)
              n635 = Equal?(x=w897, y="") -> (x = y?=w898:bool)
              n636 = call <vilib>:"Get File Extension.vi"("file"=w892) -> ("filename without extension"=w884:string, "lowercase file extension"=w885:string)  [unwired: 1 in, 8 out]
              n637 = Equal?(x=w885, y="wav") -> (x = y?=w889:bool)
              n638 = call <vilib>:"Check if File or Folder Exists.vi"("path"=w892) -> ("file or folder exists?"=w896:bool)  [unwired: 1 in, 9 out]
              n639 = Not(x=w889) -> (.not. x?=w888:bool)
              n640 = Equal?(x=w896, y=FALSE) -> (x = y?=w887:bool)
              n641 = And(x=w887, y=w888) -> (x .and. y?=w886:bool)
              n642 = case shown="FALSE" w886 {
                tunnel: w895 -> [w903 w919]
                tunnel: [w904 w920] -> w894
                tunnel: w884 -> [w901 _]
                frame False {
                  n643 = stacked-sequence {
                    tunnel: w903 -> [w909 _]
                    tunnel: [_ TRUE] -> w902
                    tunnel: w901 -> [w907 _]
                    frame #0 {
                      n644 = property on="Playlist 2" class="Listenfeld (strikt)"() -> ("Item Names"=w906:string[])  [unwired: 2 in, 2 out]
                      n645 = Initialize Array(w907, 1 ("Dimension")) -> (w908:string[])
                      n646 = Insert Into Array(array=w906, index=w909, new element=w908) -> (w905:string[])
                      n647 = property on="Playlist 2" class="Listenfeld (strikt)"("Item Names"=w905) -> ()  [unwired: 2 in, 2 out]
                    }
                    frame #1 {
                    }
                  }
                  n648 = case shown="TRUE" w902 {
                    tunnel: w903 -> [w912 w914]
                    tunnel: [w912 w913] -> w904
                    frame False {
                    }
                    frame True {
                      n649 = Increment(x=w914) -> (x+1=w913:i32)
                    }
                  }
                }
                frame True {
                  w918 = 0
                  n650 = Bundle(w919, w918) -> (w916:cluster{i32, i32})  [unwired: 1 out]
                  n651 = property on="Playlist" class="Tbl (strikt)"("Selection Size"=T5 {"Row"=1, "Column"=1} ("Größe des markierten Bereichs"), "Selection Start"=w916, "Selection Color"=u32 5 ("Markierfarbe")) -> ()  [unwired: 2 in, 2 out]
                  n652 = call "Meldung an Benutzer3"() -> ("OK"=w921:bool)  [unwired: 3 in, 8 out]
                  n653 = case shown="TRUE" w921 {
                    tunnel: w918 -> [w922 w923]
                    tunnel: [w922 w924] -> w920
                    frame False {
                    }
                    frame True {
                      n654 = Increment(x=w923) -> (x+1=w924:i32)
                    }
                  }
                }
              }
            }
          }
          event "zeile entfernen": Value Change {
            n655 = event-data() -> ()  [unwired: 7 out]
            n656 = local read "Play?"() -> (w928:bool)
            n657 = Not(x=w928) -> (.not. x?=w925:bool)
            n658 = control-ref of="Playlist"() -> (w929:refnum<vi>)
            n659 = And(x="zeile entfernen", y=w925) -> (x .and. y?=w927:bool)
            n660 = call "Zeileentfernen.vi"("Boolesch"=w927, "Referenz"=w929) -> ()
          }
          event "playlist laden": Value Change {
            n661 = event-data() -> ()  [unwired: 7 out]
          }
          event "liste löschen": Value Change {
            n662 = event-data() -> ("NewVal"=w930:bool)  [unwired: 6 out]
            n663 = case shown="TRUE" w930 {
              frame False {
              }
              frame True {
                n664 = local write "Playlist"(string[][] [] ("Playlist")) -> ()
                n665 = property on="Playlist 2" class="Listenfeld (strikt)"("Item Names"=string[] [] ("Objektnamen")) -> ()  [unwired: 2 in, 2 out]
              }
            }
          }
          event "plalist umschalten": Value Change {
            n666 = event-data() -> ("NewVal"=w933:bool)  [unwired: 6 out]
            n667 = case shown="FALSE" w933 {
              tunnel: [FALSE TRUE] -> w934
              tunnel: [TRUE FALSE] -> w935
              frame False {
              }
              frame True {
              }
            }
            n668 = property on="Playlist 2" class="Listenfeld (strikt)"("Visible"=w935) -> ()  [unwired: 2 in, 2 out]
            n669 = property on="Playlist" class="Tbl (strikt)"("Visible"=w934) -> ()  [unwired: 2 in, 2 out]
          }
          event "Musicauswählen": Value Change {
            n670 = event-data() -> ("NewVal"=w940:bool)  [unwired: 6 out]
            n671 = case shown="TRUE" w940 {
              frame False {
              }
              frame True {
                n672 = flat-sequence {
                  frame #0 {
                    n673 = Open/Create/Replace File(prompt="Please select a title." ("Eingabeaufforderung"), operation (0:open)=T2."open" ("Operation (0:Öffnen)"), access (0:read/write)=enum16{"read/write", "read-only", "write-only"}."read-only" ("Zugriff (0:Lesen/Schreiben)")) -> (refnum out=w941:refnum<file>, cancelled=w944:bool, error out=w942:errorcluster)  [unwired: 1 in, 2 out]
                    n674 = local write "Fehler (Ausgang)"(w942) -> ()
                    n675 = Refnum to Path(1:w941) -> (0:w943:path)
                    n676 = case shown="FALSE" w944 {
                      tunnel: w943 -> [w953 _]
                      tunnel: w941 -> [w948 _]
                      frame False {
                        n677 = Close File(refnum=w948) -> ()  [unwired: 1 in, 2 out]
                        n678 = call <vilib>:"Get File Extension.vi"("file"=w953) -> ("filename without extension"=w949:string, "lowercase file extension"=w952:string)  [unwired: 1 in, 8 out]
                        n679 = Equal?(x=w952, y="wav") -> (x = y?=w951:bool)
                        n680 = case shown="TRUE" w951 {
                          tunnel: w953 -> [_ w955]
                          tunnel: w949 -> [_ w954]
                          frame False {
                            n681 = call "Meldung an Benutzer7"() -> ()  [unwired: 3 in, 9 out]
                          }
                          frame True {
                            n682 = local write "Pfad"(w955) -> ()
                            "Musicanzeige" <- w954
                          }
                        }
                      }
                      frame True {
                      }
                    }
                  }
                  frame #1 {
                    "ausgewählt" <- TRUE
                  }
                }
              }
            }
          }
          event "Volume": Value Change {
            w964 = "\r"
            n683 = event-data() -> ("OldVal"=w970:i64, "NewVal"=w957:i64)  [unwired: 5 out]
            n684 = local read "min.Sound"() -> (w971:bool)
            n685 = local read "dup path"() -> (w959:path)
            n686 = Read from Text File(file (use dialog)=w959) -> (text=w958:string)  [unwired: 1 in, 5 out]
            n687 = Number To Decimal String(number=w957) -> (decimal integer string=w960:string)  [unwired: 1 out]
            n688 = Pick Line(multi-line string=w958, line index=1 ("Zeilenindex")) -> (output string=w963:string)  [unwired: 1 out]
            n689 = Pick Line(multi-line string=w958, line index=2 ("Zeilenindex")) -> (output string=w965:string)  [unwired: 1 out]
            n690 = Concatenate Strings(w960, w964, w963, w964, w965) -> (w966:string)
            n691 = case shown="TRUE" w971 {
              tunnel: w970 -> [w982 w983]
              tunnel: [w982 w984] -> w968
              frame False {
              }
              frame True {
                n692 = Less Or Equal? ("Kleiner oder gleich?")(x=w983, y=i64 10) -> (x <= y?=w986:bool)
                n693 = case shown="TRUE" w986 {
                  tunnel: [w987 11] -> w984
                  tunnel: w983 -> [w987 _]
                  frame False {
                  }
                  frame True {
                  }
                }
              }
            }
            n694 = Write to Text File(file (use dialog)=w959, text=w966) -> ()  [unwired: 1 in, 4 out]
            n695 = local read "max.Sound"() -> (w969:bool)
            n696 = case shown="TRUE" w969 {
              tunnel: w968 -> [w975 w976]
              tunnel: [w975 w977] -> w967
              frame False {
              }
              frame True {
                n697 = Greater Or Equal?(x=w976, y=80) -> (x >= y?=w978:bool)
                n698 = case shown="FALSE" w978 {
                  tunnel: [w980 79] -> w977
                  tunnel: w976 -> [w980 _]
                  frame False {
                  }
                  frame True {
                  }
                }
              }
            }
            n699 = case shown="TRUE" w971 {
              tunnel: w957 -> [_ w997]
              tunnel: [FALSE w995] -> w974
              frame False {
              }
              frame True {
                n700 = Less Or Equal? ("Kleiner oder gleich?")(x=w997, y=10) -> (x <= y?=w995:bool)
              }
            }
            n701 = case shown="TRUE" w969 {
              tunnel: w957 -> [_ w993]
              tunnel: [FALSE w991] -> w973
              frame False {
              }
              frame True {
                n702 = Greater Or Equal?(x=w993, y=80) -> (x >= y?=w991:bool)
              }
            }
            n703 = Or(x=w974, y=w973) -> (x .or. y?=w972:bool)
            n704 = case shown="TRUE" w972 {
              tunnel: w967 -> [_ w989]
              frame False {
              }
              frame True {
                n705 = local write "Volume"(w989) -> ()
                n706 = invoke on="Volume" class="Schieberegler (strikt)" method="ObjMarkieren"() -> ()  [unwired: 3 in, 3 out]
              }
            }
          }
          event "min.Sound": Value Change {
            w1004 = "\r"
            n707 = event-data() -> ("NewVal"=w998:bool)  [unwired: 6 out]
            n708 = local read "dup path"() -> (w1007:path)
            n709 = case shown="FALSE" w998 {
              tunnel: ["False" "True"] -> w1003
              frame False {
              }
              frame True {
              }
            }
            n710 = Read from Text File(file (use dialog)=w1007) -> (text=w1001:string)  [unwired: 1 in, 5 out]
            n711 = Pick Line(multi-line string=w1001, line index=0 ("Zeilenindex")) -> (output string=w1000:string)  [unwired: 1 out]
            n712 = Pick Line(multi-line string=w1001, line index=2 ("Zeilenindex")) -> (output string=w1005:string)  [unwired: 1 out]
            n713 = Concatenate Strings(w1000, w1004, w1003, w1004, w1005) -> (w1006:string)
            n714 = Write to Text File(file (use dialog)=w1007, text=w1006) -> ()  [unwired: 1 in, 4 out]
          }
          event "max.Sound": Value Change {
            w1016 = "\r"
            n715 = event-data() -> ("NewVal"=w1010:bool)  [unwired: 6 out]
            n716 = local read "dup path"() -> (w1019:path)
            n717 = case shown="TRUE" w1010 {
              tunnel: ["False" "True"] -> w1017
              frame False {
              }
              frame True {
              }
            }
            n718 = Read from Text File(file (use dialog)=w1019) -> (text=w1011:string)  [unwired: 1 in, 5 out]
            n719 = Pick Line(multi-line string=w1011, line index=0 ("Zeilenindex")) -> (output string=w1014:string)  [unwired: 1 out]
            n720 = Pick Line(multi-line string=w1011, line index=1 ("Zeilenindex")) -> (output string=w1015:string)  [unwired: 1 out]
            n721 = Concatenate Strings(w1014, w1016, w1015, w1016, w1017) -> (w1018:string)
            n722 = Write to Text File(file (use dialog)=w1019, text=w1018) -> ()  [unwired: 1 in, 4 out]
          }
          event "Sperren": Value Change {
            n723 = event-data() -> ("NewVal"=w1022:bool)  [unwired: 6 out]
            n724 = case shown="TRUE" w1022 {
              frame False {
              }
              frame True {
                n725 = local read "Deutsch?"() -> (w1028:bool)
                n726 = call "Sprachauswahl.vi"("Deutsch?"=w1028) -> ("Deutsch?"=w1025:bool)  [unwired: 10 out]
                n727 = case shown="FALSE" w1025 {
                  tunnel: ["Englisch" "Deutsch"] -> w1023
                  frame False {
                  }
                  frame True {
                  }
                }
                n728 = local read "Sicherheitsdati"() -> (w1029:path)
                n729 = Concatenate Strings("ausgewählt" ("String"), "\r", w1023) -> (w1027:string)
                n730 = Write to Text File(file (use dialog)=w1029, text=w1027) -> ()  [unwired: 1 in, 4 out]
              }
            }
          }
        }
        n731 = Wait Until Next ms Multiple(millisecond multiple=50) -> ()  [unwired: 1 out]
      }
    }
  }
  n732 = local write "anaus"(FALSE) -> ()
